vi "Vision_Right_R3.2.vi"() -> ()   [LabVIEW 2015]
uses:
  <vilib>/vision/Pattern Matching.llb/IMAQ Curve Parameters.ctl
  <vilib>/vision/Pattern Matching.llb/IMAQ Match Range Setting.ctl
  <vilib>/userdefined/High Color/IMAQdx.ctl
  <vilib>/vision/driver/NI_Vision_Acquisition_Software.lvlib
  <vilib>/vision/NI_Vision_Development_Module.lvlib
panel:
  in  "Range 0 Default\nSetting Values":T1={"Min Scale"=50.0, "Max Scale"=160.0, "Min Score"=850.0, "Lower Transition Scale"=70.0, "Upper Transition Scale"=200.0, "ROI Vertical"=2.0, "ROI Horizontal"=1.0, "Scale Cushion"=7.0, "Curve Parameters"={"Min Length"=20, "Row Search Step"=15, "Col Search Step"=15}, "Beacon Cushion (px)"=3.0, "Max Scale Diff\nfrom Main"=50.0}
  in  "Range 0 Templates":T2={"Sub - 2 File Path"=path "/home/lvuser/Beacon_Templates/Range_0/Range 0.png", "Sub Beacon Template File Path - ARRAY"=[path "/home/lvuser/Beacon_Templates/Range_1/Sub 0 - Range 1.png", path "/home/lvuser/Beacon_Templates/Range_1/Sub 1 - Range 1.png", path "/home/lvuser/Beacon_Templates/Range_1/Sub 2 - Range 1.png", path "/home/lvuser/Beacon_Templates/Range_1/Sub 3 - Range 1.png", path "/home/lvuser/Beacon_Templates/Range_1/Sub 4 - Range 1.png"]}
  in  "Correlation Score Threhsold (Range 0)":sgl=750.0
  in  "stop":bool
  in  "select (true= use advanced features\nfase= dont use)":bool
  in  "Range 3 Default\nSetting Values":T1={"Min Scale"=50.0, "Max Scale"=130.0, "Min Score"=800.0, "Lower Transition Scale"=1.0, "Upper Transition Scale"=120.0, "ROI Vertical"=4.5, "ROI Horizontal"=2.5, "Scale Cushion"=15.0, "Curve Parameters"={"Min Length"=2, "Row Search Step"=5, "Col Search Step"=5}, "Beacon Cushion (px)"=3.0, "Max Scale Diff\nfrom Main"=10.0}
  in  "Range 2 Default\nSetting Values":T1={"Min Scale"=75.0, "Max Scale"=130.0, "Min Score"=800.0, "Lower Transition Scale"=70.0, "Upper Transition Scale"=115.0, "ROI Vertical"=2.8, "ROI Horizontal"=4.0, "Scale Cushion"=17.0, "Curve Parameters"={"Min Length"=10, "Row Search Step"=10, "Col Search Step"=10}, "Beacon Cushion (px)"=7.0, "Max Scale Diff\nfrom Main"=20.0}
  in  "No Lock Default\nSetting Values":T3={"Min Scale"=25.0, "Max Scale"=125.0, "Min Score"=750.0, "Lower Transition Scale"=35.0, "Upper Transition Scale"=250.0, "ROI Vertical"=15.0, "ROI Horizontal"=15.0, "Scale Cushion"=15.0, "Curve Parameters"={"Min Length"=5, "Row Search Step"=10, "Col Search Step"=10}, "Scale Cushion 2"=15.0, "Max Scale Diff\nfrom Main"=15.0}
  in  "ROI Decay Factor (px)":dbl=50.0
  in  "ROBOT STATE\n(fwd, bwd, neither) 2":i32
  in  "Score Decay \nFactor 2":dbl=50.0
  in  "Range 1 Default\nSetting Values":T1={"Min Scale"=30.0, "Max Scale"=100.0, "Min Score"=800.0, "Lower Transition Scale"=35.0, "Upper Transition Scale"=250.0, "ROI Vertical"=0.75, "ROI Horizontal"=5.0, "Scale Cushion"=20.0, "Curve Parameters"={"Min Length"=15, "Row Search Step"=15, "Col Search Step"=15}, "Beacon Cushion (px)"=25.0, "Max Scale Diff\nfrom Main"=25.0}
  out "Next Template":T4(ring)
  out "Current Template":T4(ring)
  in  "Initial Template":T4(ring)
  in  "Range 3 Templates":T2={"Sub - 2 File Path"=path "/home/lvuser/Beacon_Templates/Range_3/5 Beacons - Range 3.png", "Sub Beacon Template File Path - ARRAY"=[path "/home/lvuser/Beacon_Templates/Range_3/Sub 0 - Range 3.png", path "/home/lvuser/Beacon_Templates/Range_3/Sub 1 - Range 3.png", path "/home/lvuser/Beacon_Templates/Range_3/Sub 2 - Range 3.png", path "/home/lvuser/Beacon_Templates/Range_3/Sub 3 - Range 3.png", path "/home/lvuser/Beacon_Templates/Range_3/Sub 4 - Range 3.png"]}
  in  "Range 2 Templates":T2={"Sub - 2 File Path"=path "/home/lvuser/Beacon_Templates/Range_2/5 Beacons - Range 2.png", "Sub Beacon Template File Path - ARRAY"=[path "/home/lvuser/Beacon_Templates/Range_2/Sub 0 - Range 2.png", path "/home/lvuser/Beacon_Templates/Range_2/Sub 1 - Range 2.png", path "/home/lvuser/Beacon_Templates/Range_2/Sub 2 - Range 2.png", path "/home/lvuser/Beacon_Templates/Range_2/Sub 3 - Range 2.png", path "/home/lvuser/Beacon_Templates/Range_2/Sub 4 - Range 2.png"]}
  in  "Range 1 Templates - LEFT":T2={"Sub - 2 File Path"=path "/home/lvuser/Beacon_Templates/Range_1/2_Beacons_Right - Range 1.png", "Sub Beacon Template File Path - ARRAY"=[path "/home/lvuser/Beacon_Templates/Range_1/Sub 0 - Range 1.png", path "/home/lvuser/Beacon_Templates/Range_1/Sub 1 - Range 1.png", path "/home/lvuser/Beacon_Templates/Range_1/Sub 2 - Range 1.png", path "/home/lvuser/Beacon_Templates/Range_1/Sub 3 - Range 1.png", path "/home/lvuser/Beacon_Templates/Range_1/Sub 4 - Range 1.png"]}
  out "Current Correlation Score":sgl=697.46326
  in  "Correlation Score Threhsold":sgl=300.0
  out "New Min Score":dbl=767.3556925455729
  out "New Low Scale":dbl=92.1760737101237
  out "New high Scale":dbl=122.1760737101237
  in  "Absolute\nMinimum Score":dbl=750.0
  in  "Absolute\nMaximum Scale":dbl=250.0
  in  "Absolute\nMinimum Scale":dbl=25.0
  in  "Score\nCushion":dbl=192.0
  in  "Avg Scale - Last":dbl=107.1760737101237
  in  "Avg Score - Last":dbl=959.3556925455729
  in  "Max Window\n for Avg":u8=3
  in  "Valid Treshold\nfor Lock":i16=3
  out "Current  Score":sgl=956.6209
  out "Current  Scale":sgl=107.15872
  out "Current Valid?":bool=TRUE
  out "Beacon - Scales":sgl[](array[numeric])=[106.93824, 100.57165, 104.69414, 100.46582, 110.0]
  out "beacon - Scores":sgl[](array[numeric])=[992.1048, 981.1018, 1000.0, 999.00995, 773.5499]
  out "Beacons Found":bool[](array[boolean])=[TRUE, TRUE, TRUE, TRUE, TRUE]
  in  "Horiztonall Beacon \nCushion (pixels)":sgl=7.0
  out "Tracking Info":T5={"Lock"=TRUE, "Current Valid"=TRUE, "Current Template"=enum."Range 2", "Tracking Coordinates"={"X"=158.2768096923828, "Y"=119.25008392333984}, "Setting Values"={"Min Score"=767.3556925455729, "Min Scale"=92.1760737101237, "Max Scale"=122.1760737101237, "Curve Parameters"={"Min Length"=10, "Row Search Step"=10, "Col Search Step"=10}}}
  out "dT":u32=420
  out "Avg Scale":dbl=107.1760737101237
  out "Avg Score":dbl=959.3556925455729
  out "Current Search Settings":T8={"Curve Parameters"={"Extraction Mode"=1, "Edge Threshold"=200, "Edge Filter Size"=0, "Min Length"=10, "Row Search Step Size"=10, "Col Search Step Size"=10, "Max Endpoint Gap"=4, "Closed"=TRUE, "Subpixel"=TRUE}, "Match Mode"={"Rotation"=FALSE, "Scale"=TRUE, "Occlusion"=TRUE, "Reserved"=FALSE, "Reserved"=FALSE, "Reserved"=FALSE}, "Range Settings"=[{"Match Constraints"=0, "Min"=-2.0, "Max"=2.0}, {"Match Constraints"=1, "Min"=92.1760737101237, "Max"=122.1760737101237}, {"Match Constraints"=2, "Min"=0.0, "Max"=20.0}], "Number of Matches"=1, "Minimum Match Score"=767.3557, "SubPixel Accuracy"=TRUE, "Adv. Geometric Match Options 2"=[{"Setup Data Item"=20, "Item Value"=0.0}, {"Setup Data Item"=22, "Item Value"=1.0}]} {"Curve Parameters"."Extraction Mode" items=["Normal", "Uniform Regions"]; "Curve Parameters"."Edge Filter Size" items=["Fine", "Normal", "Contour Tracing"]; "Curve Parameters"."Max Endpoint Gap" min=0; "Curve Parameters"."Col Search Step Size" min=1 max=255 step=1; "Curve Parameters"."Row Search Step Size" min=1 max=255 step=1; "Curve Parameters"."Min Length" min=0; "Curve Parameters"."Edge Threshold" min=1 max=350 step=1; "Range Settings"."Max" format="%.2f"; "Range Settings"."Min" format="%.2f"; "Range Settings"."Match Constraints" items=["Rotation Angle (degrees)", "Scale Factor (%)", "Occlusion (%)"]}
  out "Valid Scale History":dbl[](array[numeric])=[107.15872192382812, 107.20863342285156, 107.1608657836914, 106.95974731445312, 107.13298034667969, 106.9737319946289, 107.18673706054688, 106.71354675292969, 106.60578918457031, 106.39472961425781, 106.54171752929688, 105.94715118408203, 107.21797943115234, 106.39393615722656, 106.02467346191406, 106.8507308959961, 106.52826690673828, 105.7506103515625, 107.49342346191406] format="%#_13g"
  out "Valid Score History":dbl[](array[numeric])=[956.6209106445312, 957.1117553710938, 964.3344116210938, 965.7691650390625, 956.08837890625, 958.0139770507812, 954.0676879882812, 955.1304931640625, 955.5637817382812, 955.6036376953125, 955.892822265625, 972.4268798828125, 965.9573974609375, 966.6751098632812, 968.4617309570312, 967.2622680664062, 967.345947265625, 978.3862915039062, 966.6702880859375] format="%#_13g"
  out "Valid Beacon History - in":bool[](array[boolean])=[TRUE, TRUE, TRUE, TRUE, TRUE, TRUE, TRUE, TRUE, TRUE, TRUE, TRUE, TRUE, TRUE, TRUE, TRUE, TRUE, TRUE, TRUE, TRUE]
  out "Startup Flag":bool
  out "Lock Status":bool=TRUE
  out "Y Coordinates":sgl[](array[numeric])=[117.82886, 117.06131, 119.28133, 118.96902, 113.5]
  out "X Coordinates":sgl[](array[numeric])=[55.56325, 105.59997, 158.00548, 202.0866, 251.0]
  out "Right Image out":T9(plugin-control)
  in  "History Size":i32=19
  in  "INITIAL Search Settings":T8={"Curve Parameters"={"Extraction Mode"=1, "Edge Threshold"=200, "Edge Filter Size"=0, "Min Length"=15, "Row Search Step Size"=10, "Col Search Step Size"=10, "Max Endpoint Gap"=4, "Closed"=TRUE, "Subpixel"=TRUE}, "Match Mode"={"Rotation"=TRUE, "Scale"=TRUE, "Occlusion"=TRUE, "Reserved"=FALSE, "Reserved"=FALSE, "Reserved"=FALSE}, "Range Settings"=[{"Match Constraints"=0, "Min"=-10.0, "Max"=1.0}, {"Match Constraints"=1, "Min"=25.0, "Max"=150.0}, {"Match Constraints"=2, "Min"=0.0, "Max"=20.0}], "Number of Matches"=1, "Minimum Match Score"=750.0, "SubPixel Accuracy"=TRUE, "Adv. Geometric Match Options 2"=[{"Setup Data Item"=20, "Item Value"=0.0}, {"Setup Data Item"=22, "Item Value"=1.0}]} {"Curve Parameters"."Extraction Mode" items=["Normal", "Uniform Regions"]; "Curve Parameters"."Edge Filter Size" items=["Fine", "Normal", "Contour Tracing"]; "Curve Parameters"."Max Endpoint Gap" min=0; "Curve Parameters"."Col Search Step Size" min=1 max=255 step=1; "Curve Parameters"."Row Search Step Size" min=1 max=255 step=1; "Curve Parameters"."Min Length" min=0; "Curve Parameters"."Edge Threshold" min=1 max=350 step=1; "Range Settings"."Max" format="%.2f"; "Range Settings"."Min" format="%.2f"; "Range Settings"."Match Constraints" items=["Rotation Angle (degrees)", "Scale Factor (%)", "Occlusion (%)"]; "Adv. Geometric Match Options 2"."Setup Data Item" items=["Curve Extraction Mode", "Curve Edge Threshold", "Curve Edge Filter Size", "Min Curve Length", "Curve Row Search Step Size", "Curve Col Search Step Size", "Curve Max Endpoint Gap", "Extract Closed Curves", "Enable Subpixel Curve Extraction", "Enable Correlation Score", "Enable Subpixel Accuracy", "Subpixel Iterations", "Subpixel Tolerance", "Initial Match List Length", "Enable Target Template Curve Score", "Min Match Separation Distance", "Min Match Separation Angle", "Min Match Separation Scale", "Max Match Overlap", "Enable Coarse Result", "Enable Calibration Support", "Enable Contrast Reversal", "Search Strategy", "Refinement Match Factor", "Subpixel Match Factor"]}
  # "ROI Factore (per Template)"
  # "Template Transition Scales"
  # "Search Parameter Limits"
  # "TEMPLATE FILE PATHS"
  # "Config"
  # "Initial Settings"
  # "Range"
  # "Range"
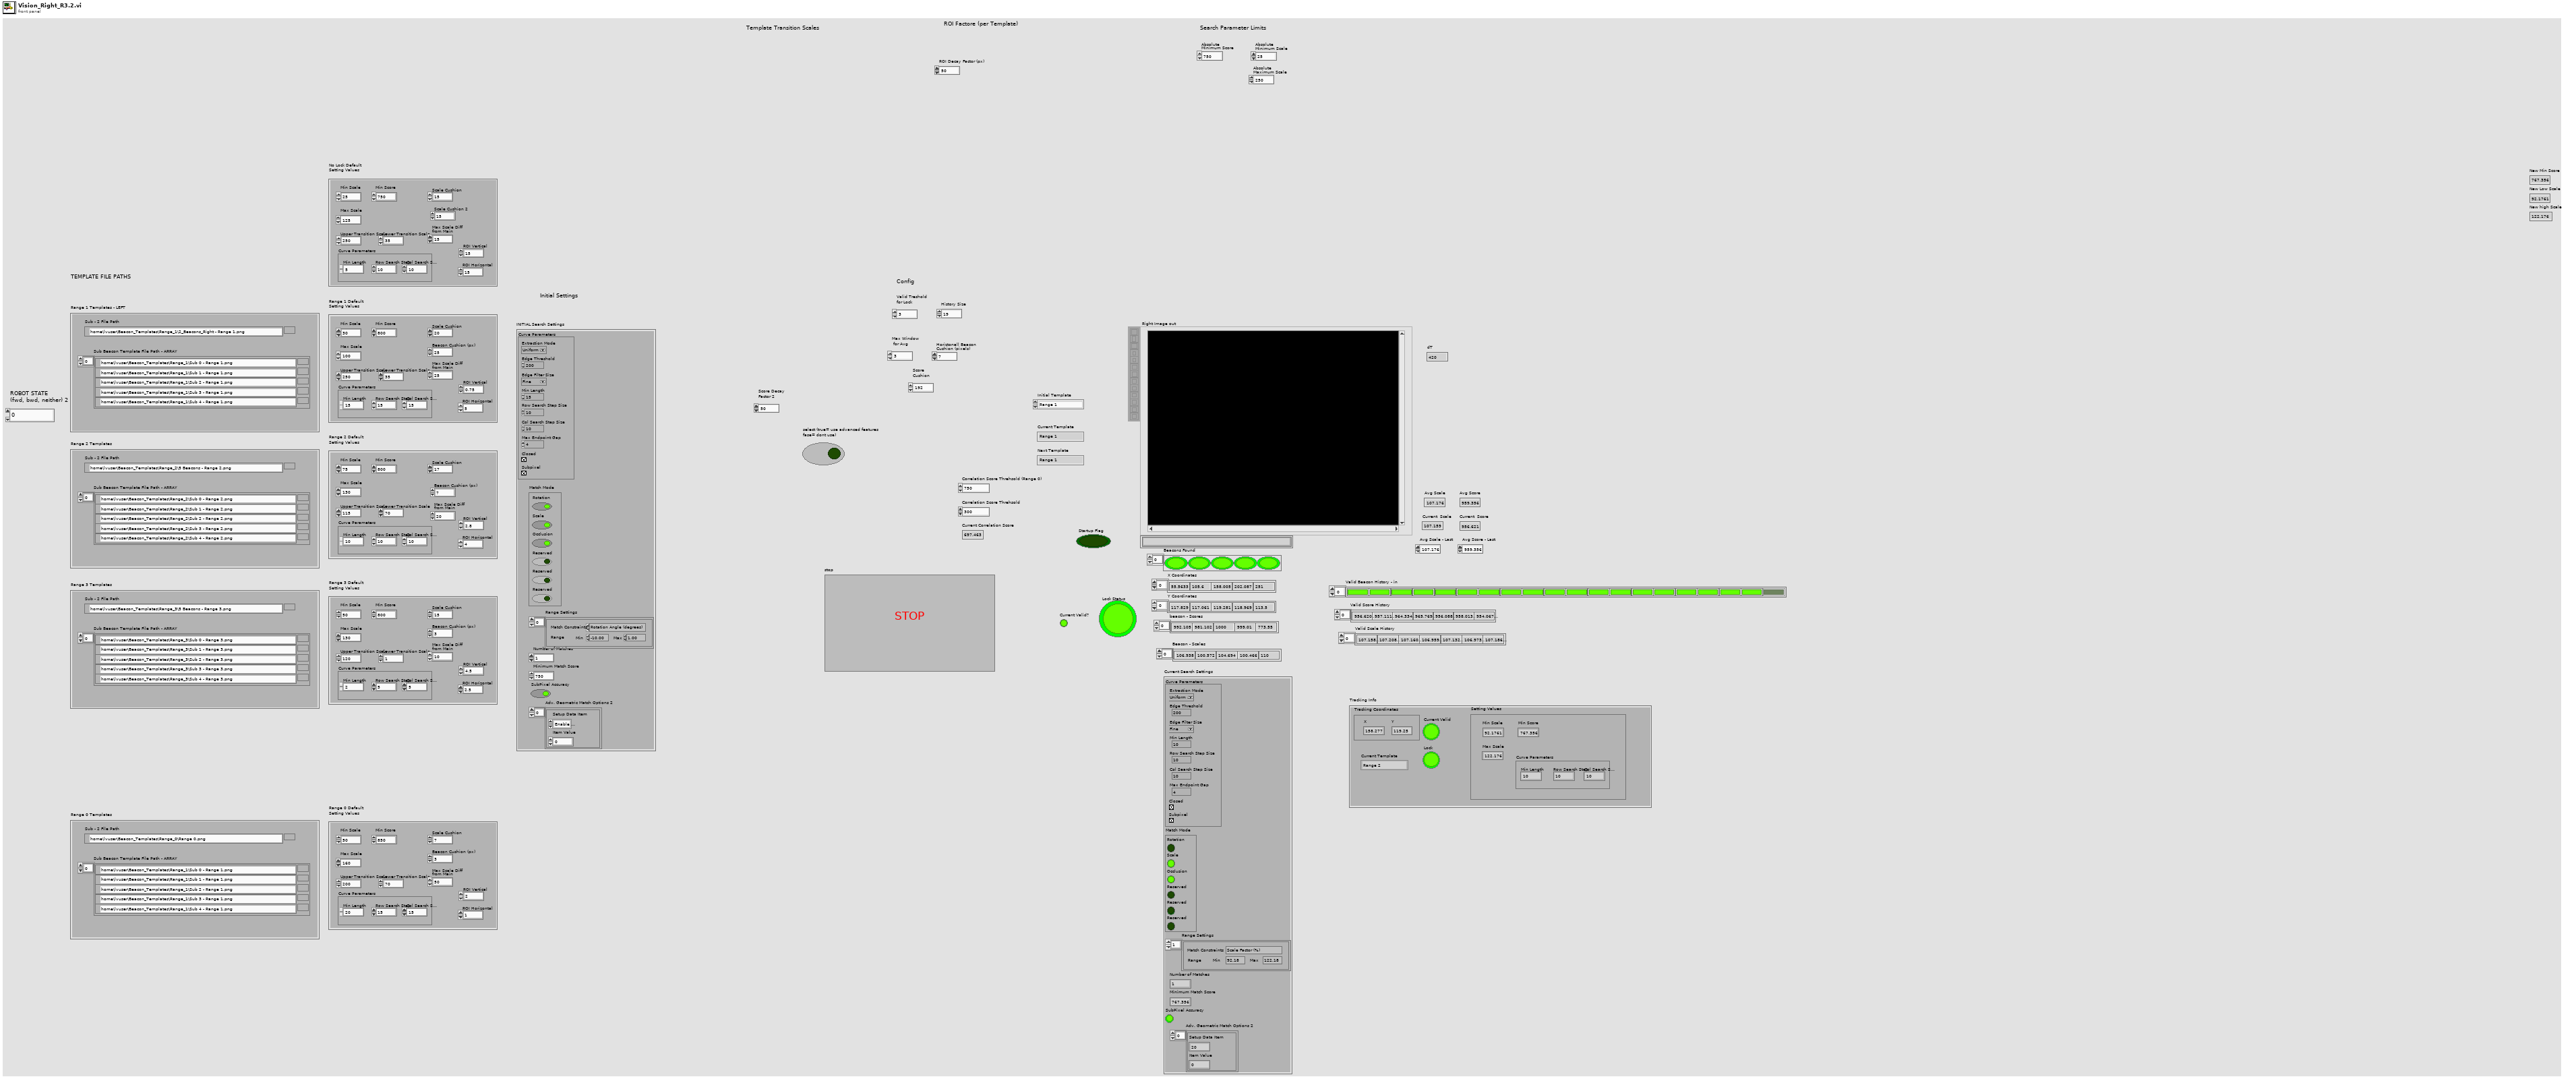
[diagram p1: front panel]
types:
  T1 = cluster{"Min Scale":dbl, "Max Scale":dbl, "Min Score":dbl, "Lower Transition Scale":sgl, "Upper Transition Scale":sgl, "ROI Vertical":dbl, "ROI Horizontal":dbl, "Scale Cushion":dbl, "Curve Parameters":cluster{"Min Length":i32, "Row Search Step":i32, "Col Search Step":i32}, "Beacon Cushion (px)":dbl, "Max Scale Diff\nfrom Main":dbl}
  T2 = cluster{"Sub - 2 File Path":path, "Sub Beacon Template File Path - ARRAY":path[]}
  T3 = cluster{"Min Scale":dbl, "Max Scale":dbl, "Min Score":dbl, "Lower Transition Scale":sgl, "Upper Transition Scale":sgl, "ROI Vertical":dbl, "ROI Horizontal":dbl, "Scale Cushion":dbl, "Curve Parameters":cluster{"Min Length":i32, "Row Search Step":i32, "Col Search Step":i32}, "Scale Cushion 2":dbl, "Max Scale Diff\nfrom Main":dbl}
  T4 = enum16{"Range 1", "Range 2", "Range 3", "Range 0"}
  T5 = cluster{"Lock":bool, "Current Valid":bool, "Current Template":enum16{"Range 1", "Range 2", "Range 3", "Range 0"}, "Tracking Coordinates":cluster{"X":dbl, "Y":dbl}, "Setting Values":cluster{"Min Score":dbl, "Min Scale":dbl, "Max Scale":dbl, "Curve Parameters":cluster{"Min Length":i32, "Row Search Step":i32, "Col Search Step":i32}}}
  T6 = typedef "IMAQ Curve Parameters.ctl" = cluster{"Extraction Mode":u32, "Edge Threshold":i32, "Edge Filter Size":u32, "Min Length":i32, "Row Search Step Size":i32, "Col Search Step Size":i32, "Max Endpoint Gap":i32, "Closed":bool, "Subpixel":bool}
  T7 = typedef "IMAQ Match Range Setting.ctl" = cluster{"Match Constraints":u32, "Min":dbl, "Max":dbl}
  T8 = cluster{"Curve Parameters":T6, "Match Mode":cluster{"Rotation":bool, "Scale":bool, "Occlusion":bool, "Reserved":bool, "Reserved":bool, "Reserved":bool}, "Range Settings":T7[], "Number of Matches":i32, "Minimum Match Score":sgl, "SubPixel Accuracy":bool, "Adv. Geometric Match Options 2":cluster{"Setup Data Item":u16, "Item Value":dbl}[]}
  T9 = typedef "IMAQ Image.ctl" = refnum<image>
  T10 = typedef "IMAQdx.ctl" = refnum<k21>
  T11 = typedef "Image Type" = u32
  T12 = typedef "ROI Descriptor" = cluster{"Global Rectangle":i32[], "Contours":cluster{"ID":enum32{"External", "Internal"}, "Type":u32, "Coordinates":i32[]}[]}
  T13 = typedef "IMAQ GM Match Report.ctl" = cluster{"Position":cluster{"x":sgl, "y":sgl}, "Angle":sgl, "Scale":sgl, "Score":sgl, "Bounding Box":cluster{"x":sgl, "y":sgl}[], "Contrast Reversed":bool, "Occlusion %":sgl, "Template Target Curve Score":sgl, "Target Template Curve Score":sgl, "Correlation Score":sgl}
  T14 = cluster{"Matches[0]":T13, "Matches[1]":T13, "Matches[2]":T13, "Matches[3]":T13, "Matches[4]":T13, "Matches[5]":T13, "Matches[6]":T13, "Matches[7]":T13, "Matches[8]":T13}
  T15 = cluster{"Bounding Box[0]":cluster{"x":sgl, "y":sgl}, "Bounding Box[1]":cluster{"x":sgl, "y":sgl}, "Bounding Box[2]":cluster{"x":sgl, "y":sgl}, "Bounding Box[3]":cluster{"x":sgl, "y":sgl}, "Bounding Box[4]":cluster{"x":sgl, "y":sgl}, "Bounding Box[5]":cluster{"x":sgl, "y":sgl}, "Bounding Box[6]":cluster{"x":sgl, "y":sgl}, "Bounding Box[7]":cluster{"x":sgl, "y":sgl}, "Bounding Box[8]":cluster{"x":sgl, "y":sgl}}
  T16 = cluster{"Matches (Geometric Matching 1)[0]":T13, "Matches (Geometric Matching 1)[1]":T13, "Matches (Geometric Matching 1)[2]":T13, "Matches (Geometric Matching 1)[3]":T13, "Matches (Geometric Matching 1)[4]":T13, "Matches (Geometric Matching 1)[5]":T13, "Matches (Geometric Matching 1)[6]":T13, "Matches (Geometric Matching 1)[7]":T13, "Matches (Geometric Matching 1)[8]":T13}
  T17 = cluster{"Min Length":i32, "Row Search Step":i32, "Col Search Step":i32}
  T18 = cluster{"Extraction Mode":u32, "Edge Threshold":i32, "Edge Filter Size":u32, "Min Length":i32, "Row Search Step":i32, "Col Search Step":i32, "Max Endpoint Gap":i32, "Closed":bool, "Subpixel":bool}
  T19 = typedef "IMAQ Rectangle" = cluster{"Left":i32, "Top":i32, "Right":i32, "Bottom":i32, "Rotation":dbl}
  T20 = cluster{"Min Length":i32, "Row Search Step Size":i32, "Col Search Step Size":i32}
  T21 = cluster{"Min Score":dbl, "Min":dbl, "Max":dbl, cluster{"Min Length":i32, "Row Search Step Size":i32, "Col Search Step Size":i32}}
  T22 = cluster{bool, bool, "Initial Template":enum16{"Range 1", "Range 2", "Range 3", "Range 0"}, "Position":cluster{"x":dbl, "y":dbl}, cluster{"Min Score":dbl, "Min":dbl, "Max":dbl, cluster{"Min Length":i32, "Row Search Step Size":i32, "Col Search Step Size":i32}}}
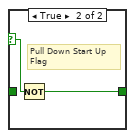
[diagram p2: hidden frame]
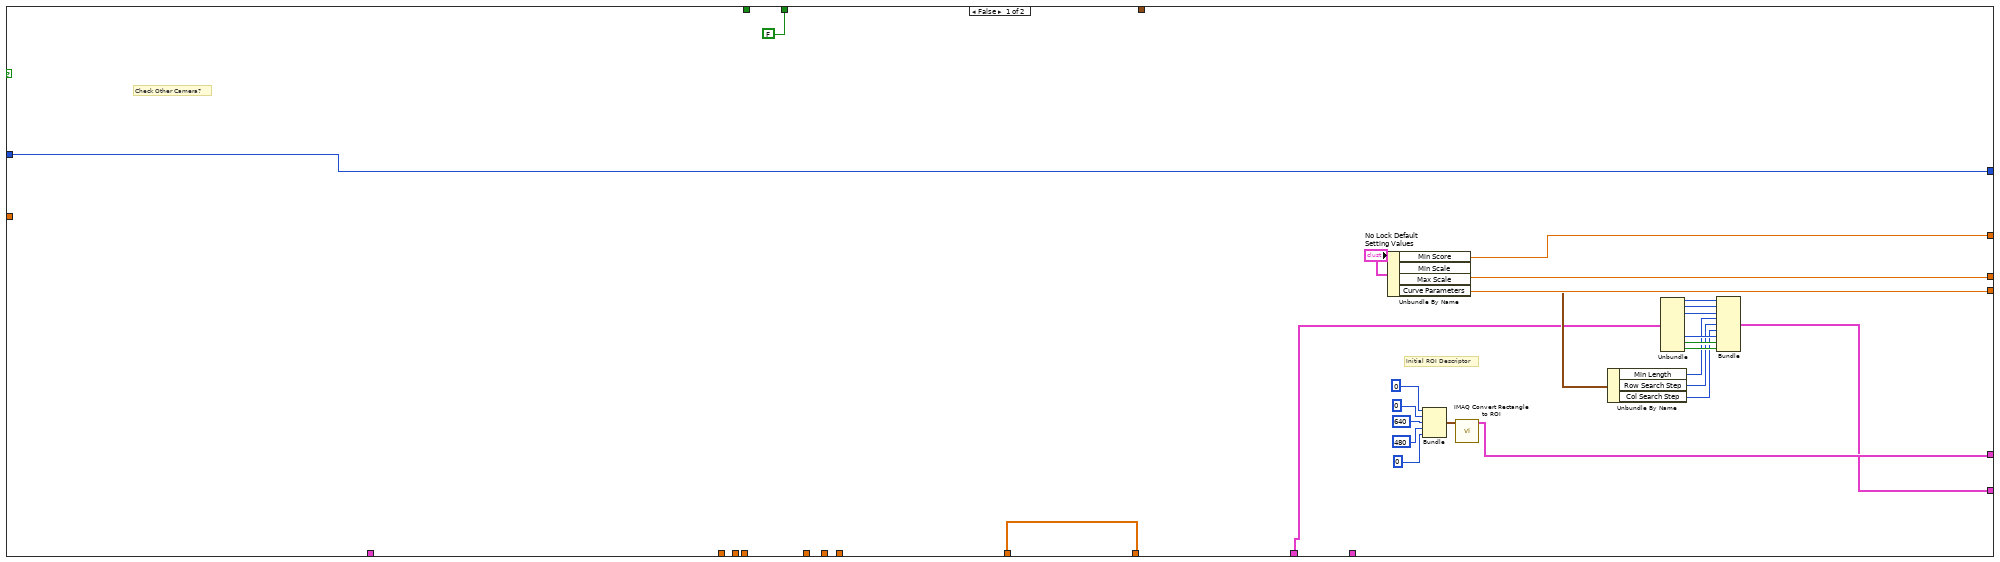
[diagram p3: hidden frame]
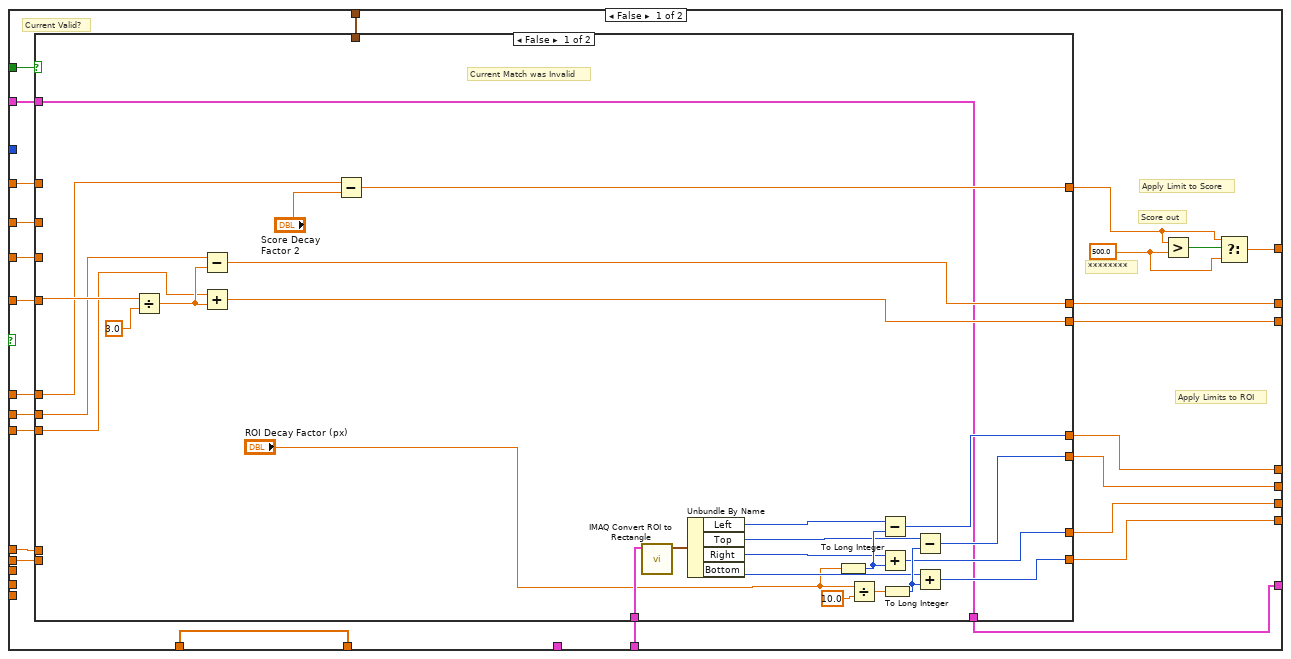
[diagram p4: hidden frame]
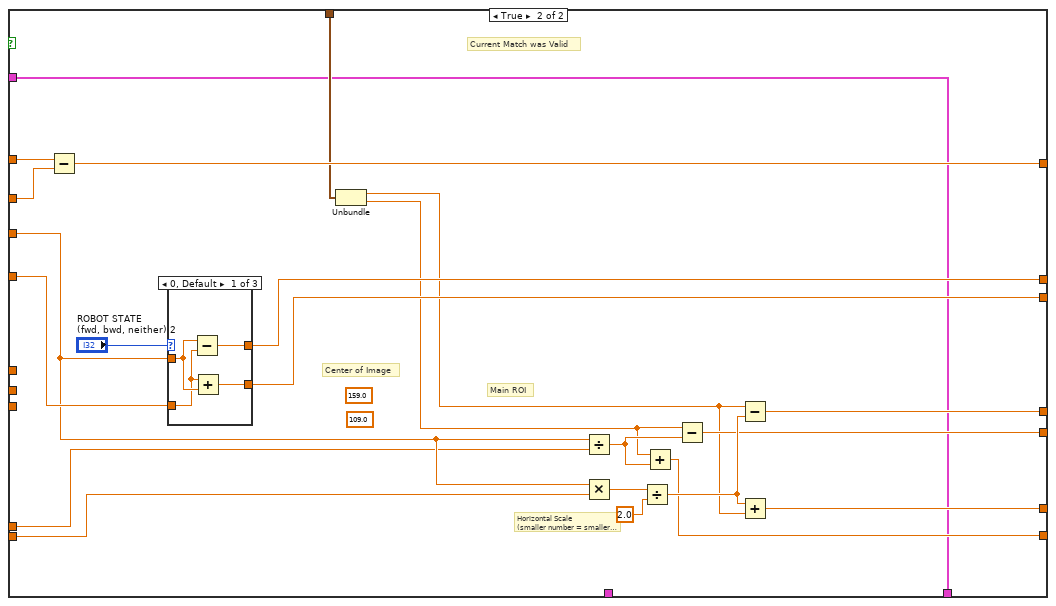
[diagram p5: hidden frame]
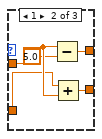
[diagram p6: hidden frame]
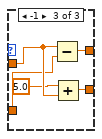
[diagram p7: hidden frame]
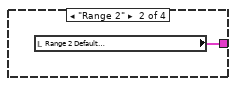
[diagram p8: hidden frame]
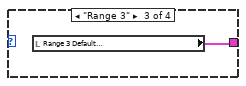
[diagram p9: hidden frame]
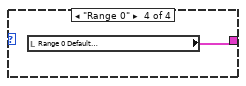
[diagram p10: hidden frame]
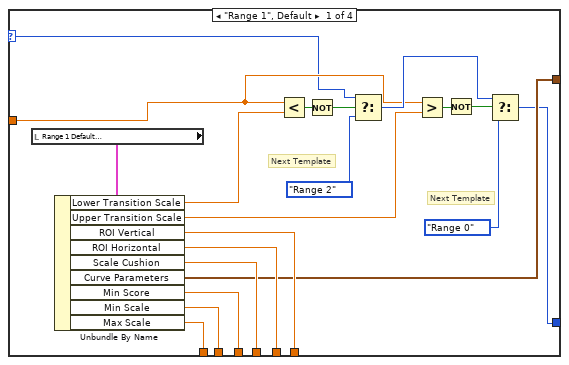
[diagram p11: hidden frame]
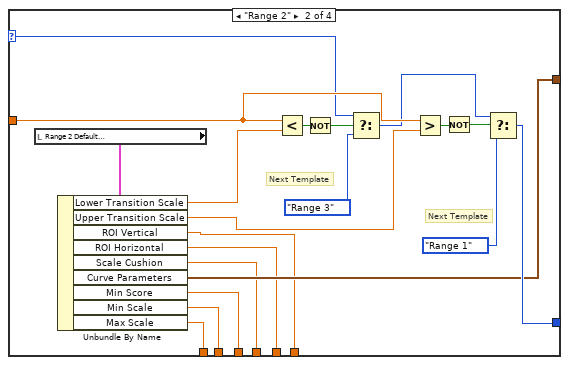
[diagram p12: hidden frame]
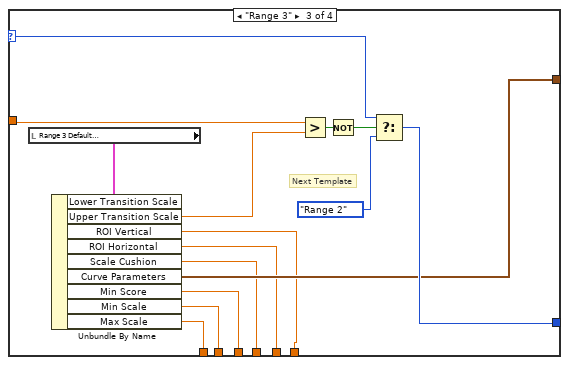
[diagram p13: hidden frame]
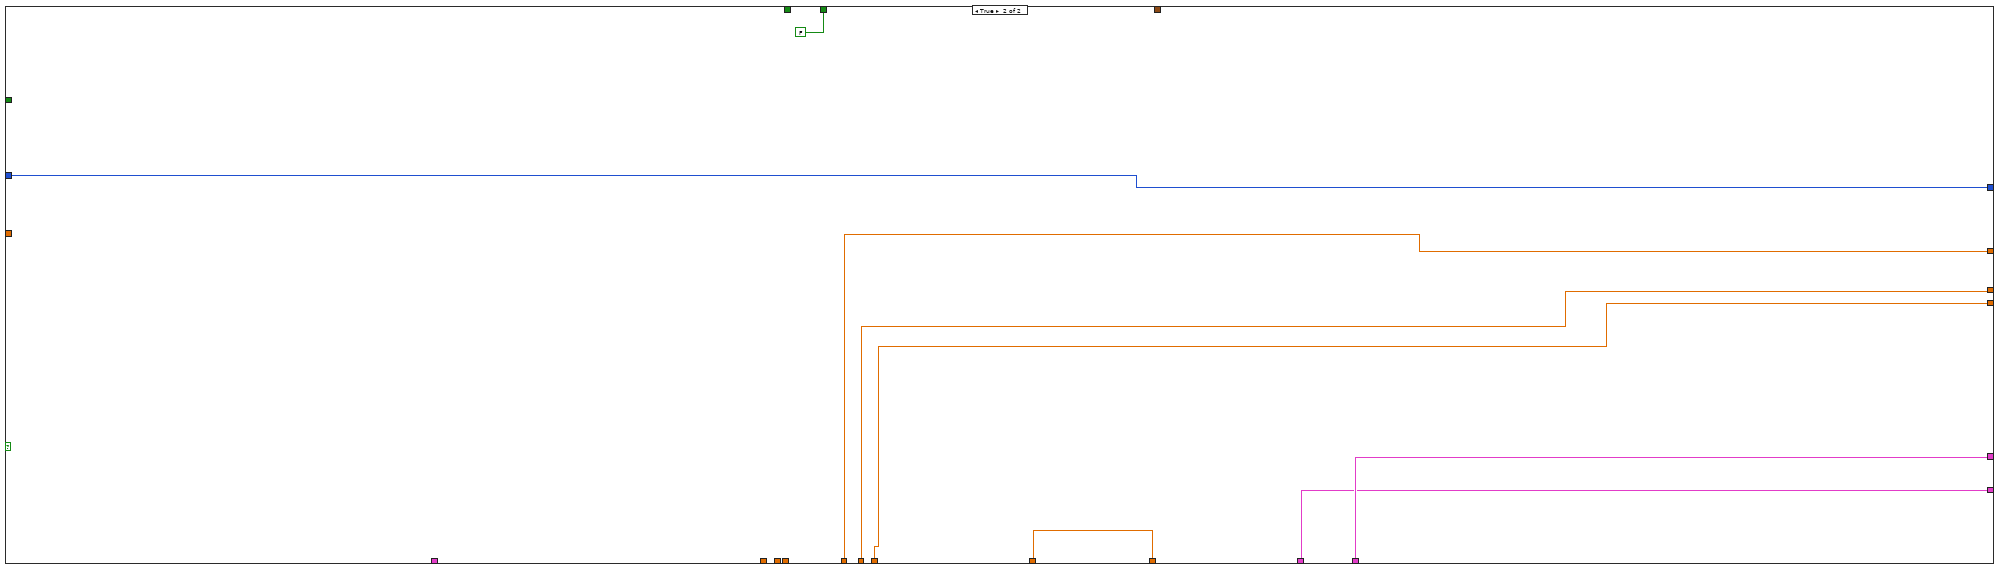
[diagram p14: hidden frame]
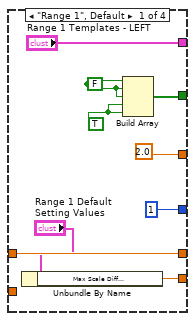
[diagram p15: hidden frame]
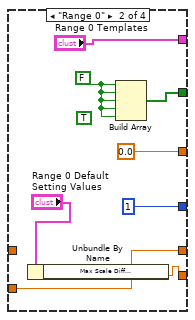
[diagram p16: hidden frame]
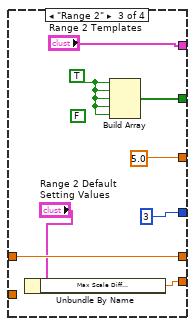
[diagram p17: hidden frame]
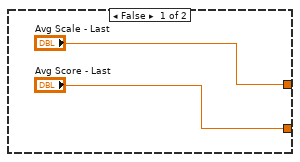
[diagram p18: hidden frame]
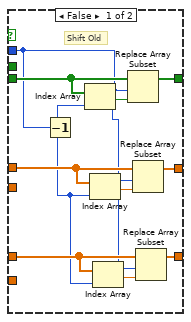
[diagram p20: hidden frame]
diagram:
  n1 = flat-sequence {
    tunnel: [w38] -> w16
    tunnel: ["INITIAL Search Settings"] -> w15
    tunnel: ["Initial Template"] -> w14
    tunnel: [TRUE] -> w13
    tunnel: [w35] -> w12
    tunnel: [w34] -> w11
    tunnel: [w33] -> w10
    tunnel: [w32] -> w9
    tunnel: [w31] -> w8
    tunnel: ["History Size"] -> w7
    tunnel: [750.0] -> w6
    tunnel: [100.0] -> w5
    tunnel: [w19] -> w4
    tunnel: [w18] -> w3
    tunnel: [w17] -> w2
    tunnel: w16 -> [w64]
    tunnel: w15 -> [w63]
    tunnel: w14 -> [w62]
    tunnel: w13 -> [w61]
    tunnel: w12 -> [w57]
    tunnel: w11 -> [w54]
    tunnel: w10 -> [w60]
    tunnel: w9 -> [w59]
    tunnel: w8 -> [w58]
    tunnel: w7 -> [w56]
    tunnel: w6 -> [_]
    tunnel: w5 -> [_]
    tunnel: w4 -> [w53]
    tunnel: w3 -> [w52]
    tunnel: w2 -> [w51]
    tunnel: [w50] -> w1
    tunnel: w1 -> [w825]
    frame #0 {
      w24 = "[NIIMAQ_HEADER]\nType = 2\nVersion = 8\n\n[CAMERA_DATA]\nAcquisitionAttributes::Bayer::Algorithm = \"Bilinear\"\nAcquisitionAttributes::Bayer::GainB = \"1\"\nAcquisitionAttributes::Bayer::GainG = \"1\"\nAcquisitionAttributes::Bayer::GainR = \"1\"\nAcquisitionAttributes::Bayer::Pattern = \"Use hardware value\"\nAcquisitionAttributes::BitsPerPixel = \"Use hardware value\"\nAcquisitionAttributes::IgnoreFirstFrame = \"false\"\nAcquisitionAttributes::ImageDecoderCopyMode = \"Auto\"\nAcquisitionAttributes::OutputImageType = \"Auto\"\nAcquisitionAttributes::OverwriteMode = \"Get Newest\"\nAcquisitionAttributes::PixelSignedness = \"Use hardware value\"\nAcquisitionAttributes::ReceiveTimestampMode = \"None\"\nAcquisitionAttributes::ShiftPixelBits = \"false\"\nAcquisitionAttributes::SwapPixelBytes = \"false\"\nAcquisitionAttributes::Timeout = \"5000\"\nAcquisitionAttributes::VerticalMirror = \"false\"\nAcquisitionAttributes::VideoMode = \"320x240 YUY2 30.00fps\"\nCameraAttributes::BacklightCompensation::Mode = \"Manual\"\nCameraAttributes::BacklightCompensation::Value = \"false\"\nCameraAttributes::Brightness::Mode = \"UnknownEnumValue\"\nCameraAttributes::Brightness::Value = \"133\"\nCameraAttributes::Contrast::Mode = \"Manual\"\nCameraAttributes::Contrast::Value = \"0\"\nCameraAttributes::Exposure::Mode = \"Auto\"\nCameraAttributes::Focus::Mode = \"Auto\"\nCameraAttributes::Pan::Mode = \"Manual\"\nCameraAttributes::Pan::Value = \"0\"\nCameraAttributes::Saturation::Mode = \"Manual\"\nCameraAttributes::Saturation::Value = \"103\"\nCameraAttributes::Sharpness::Mode = \"Manual\"\nCameraAttributes::Sharpness::Value = \"25\"\nCameraAttributes::Tilt::Mode = \"Manual\"\nCameraAttributes::Tilt::Value = \"0\"\nCameraAttributes::WhiteBalance::Mode = \"Auto\"\nCameraAttributes::Zoom::Mode = \"Manual\"\nCameraAttributes::Zoom::Value = \"0\"\n"  # Attributes
      w45 = T11 0 items=["Grayscale (U8)", "Grayscale (I16)", "Grayscale (SGL)", "Complex (CSG)", "RGB (U32)", "HSL (U32)", "RGB (U64)", "Grayscale (U16)"] ("Image Type")
      # "avg start scale"
      # "Score History"
      # "Scale History"
      # "Valid Match History\n(main beacon)"
      # "Template State"
      # "Search Parameters"
      # "StartUp = True"
      # "Initial ROI Descriptor"
      # "INITIALIZE"
      n2 = call <vilib>:"IMAQdx Open Camera.vi"("Session In"=T10 "cam0") -> ("error out"=w22:errorcluster, "Session Out"=w23:T10)  [unwired: 2 in, 7 out]
      n3 = call <vilib>:"IMAQdx Read Attributes From String.vi"("error in"=w22, "Attributes String In"=w24, "Session In"=w23) -> ("error out"=w21:errorcluster, "Session Out"=w20:T10)  [unwired: 7 out]
      n4 = Bundle(0, 0, 640, 480, 0) -> (w44:cluster{i32, i32, i32, i32, i32})  [unwired: 1 in]
      n5 = call "IMAQ Convert Rectangle to ROI"("Rectangle"=w44) -> ("ROI Descriptor"=w38:T12)  [unwired: 8 in, 1 out]
      n6 = call "IMAQ Create"("Image Name"="Left_Image", "Image Type"=w45) -> ("New Image"=w35:T9, "error out"=w34:errorcluster)  [unwired: 3 in]
      n7 = Initialize Array(FALSE, "History Size") -> (w33:bool[])
      n8 = Initialize Array(0.0, "History Size") -> (w31:dbl[])
      n9 = Initialize Array(0.0, "History Size") -> (w32:dbl[])
      n10 = call <vilib>:"IMAQdx Configure Grab.vi"("error in"=w21, "Session In"=w20) -> ("error out"=w17:errorcluster, "Session Out"=w19:T10)  [unwired: 8 in]
      n11 = call "IMAQ Create"("Image Name"="Original") -> ("New Image"=w18:T9)  [unwired: 4 in, 1 out]
    }
    frame #1 {
      # "Avg Scale"
      # "Avg Score"
      # "Score History"
      # "Scale History"
      # "Valid Match History\n(main beacon)"
      # "Sub Beacon Search Array"
      # "StartUp = True"
      # "Template State"
      # "Search Parameters"
      # "ROI"
      n12 = call "Tick Count"() -> ("Tick Count(mSec)"=w55:u32)
      n13 = while {
        shift-right: [w77] -> _
        shift-left: w64 -> [w91]
        shift-right: [w87] -> _
        shift-left: w63 -> [w92]
        shift-right: [w76] -> _
        shift-left: w62 -> [w79]
        shift-right: [w74] -> _
        shift-left: w61 -> [w75]
        shift-right: [w83] -> _
        shift-left: w60 -> [w84]
        shift-right: [w73] -> _
        shift-left: w59 -> [w82]
        shift-right: [w80] -> _
        shift-left: w58 -> [w81]
        shift-right: [w86] -> _
        shift-left: w57 -> [w93]
        tunnel: w56 -> [w98]
        shift-right: [w96] -> _
        shift-left: w55 -> [w97]
        tunnel: w54 -> [w85]
        tunnel: w53 -> [w72]
        tunnel: w52 -> [w71]
        tunnel: w51 -> [w70]
        tunnel: [w67] -> w50
        stop <- "stop" stop-if-true
        n14 = call "Tick Count2"() -> ("Tick Count(mSec)"=w96:u32)
        n15 = Subtract(x=w96, y=w97) -> (x-y=→"dT":u32)
        n16 = flat-sequence {
          tunnel: [w106] -> w89
          tunnel: [w105] -> w94
          tunnel: w93 -> [w105]
          tunnel: [w105] -> w86
          tunnel: w85 -> [_]
          tunnel: w72 -> [w104]
          tunnel: w71 -> [w103]
          tunnel: w70 -> [w102]
          tunnel: [w101] -> w69
          tunnel: [w100] -> w68
          tunnel: [w99] -> w66
          tunnel: w79 -> [w110]
          tunnel: w84 -> [w223]
          tunnel: w82 -> [w222]
          tunnel: w81 -> [w221]
          tunnel: w98 -> [_]
          tunnel: w94 -> [w121]
          tunnel: w92 -> [w122]
          tunnel: w91 -> [w124]
          tunnel: [w190] -> w90
          tunnel: w89 -> [w179]
          tunnel: [w179] -> w88
          tunnel: [w178] -> w83
          tunnel: [w146] -> _
          tunnel: [w177] -> w80
          tunnel: w75 -> [w143]
          tunnel: [w148] -> w78
          tunnel: [w149] -> w77
          tunnel: [w148] -> w76
          tunnel: [w142] -> w74
          tunnel: [w147] -> w73
          tunnel: w69 -> [w116]
          tunnel: w68 -> [w115]
          tunnel: [w114] -> w67
          tunnel: w66 -> [w114]
          tunnel: w90 -> [w822]
          tunnel: w88 -> [w823]
          tunnel: [w822] -> w87
          tunnel: [w821] -> _
          tunnel: w78 -> [w821]
          frame #0 {
            # "Aquire Image"
            n17 = shared-variable "RT myRIO Target - Overlord\\Localization_Variables_r0.lvlib\\Right Servo Angle_Current"() -> (w106:dbl)  [unwired: 1 in, 1 out]
            n18 = call <vilib>:"IMAQdx Grab2.vi"("error in"=w102, "Image In"=w103, "Session In"=w104) -> ("error out"=w100:errorcluster, "Image Out"=w101:T9, "Session Out"=w99:T10)  [unwired: 5 in, 1 out]
          }
          frame #1 {
            (unwired) T4."Range 1" ("Initial Template 2")
            w134 = 6 items=["Red", "Green", "Blue", "Hue", "Saturation", "Luminance", "Value", "Intensity"] ("Color Plane")
            w193 = u32 1 ("index")
            # "Tracking Position"
            # "ROI center"
            # "Add mode when CLose to look for all individual beacons with full ROI"
            # "Service Start Up Flag"
            # "Change States?"
            # "Next Template"
            # "Max Scale"
            # "Min Scale"
            # "Min Score"
            # "Curve p"
            # "ROI"
            # "Current Scale Range"
            # "Current Min Score"
            # "Avg Score"
            # "Avg Scale"
            # "Startup?"
            # "********** Look into False case **********"
            # "SUm # of Sub-Beacons Found, Check if Enoough\nto be considered Valid"
            # "Update Tracking Coordinates"
            # "Next Settings"
            # "Current Settings"
            # "Current Min\n& Max Scale"
            # "Scale"
            # "Min Score"
            # "Lower Scale"
            # "Upper Scale"
            # "Min Score out"
            # "Score History"
            # "Min Required to use avarage"
            # "Scale History"
            # "History Size"
            # "Calculate Average Score/Scale"
            # "****# of previous in history that must be true\nin order for position to be considered \"locked\""
            # "Scale History"
            # "Score History"
            # "Valid History"
            # "Update History Data"
            # "1 Match FOund?"
            # "# of Sub Beacons"
            # "Sub Beacons to Search For"
            # "# Sub Beacons to Find in\norder to be valid"
            # "Template Filepath & Sub Beacon Array"
            # "Select Current Template Config"
            # "Pattern Match to Current Template"
            # "Apply FIltering"
            n19 = call "IMAQ ImageBorderSize"("Get/Set Status? (Set)"=TRUE, "Image"=w116, "Image border size in"=13 ("Border Size"), "error in (no error)"=w115) -> ("Image Out"=w133:T9, "error out"=w137:errorcluster)  [unwired: 1 out]
            n20 = call "IMAQ ExtractSingleColorPlane"("Color Plane"=w134, "error in (no error)"=w137, "Image Src"=w133) -> ("error out"=w132:errorcluster, "Image Dst Out"=w130:T9)  [unwired: 1 in, 6 out]
            n21 = call "IMAQ Convolute"("Kernel"=sgl[][] [[1.0, 2.0, 1.0], [2.0, 4.0, 2.0], [1.0, 2.0, 1.0]], "Divider (kernel sum)"=sgl 9.0 ("Divider"), "error in (no error)"=w132, "Image Src"=w130) -> ("error out"=w129:errorcluster, "Image Dst Out"=w126:T9)  [unwired: 3 in, 3 out]
            n22 = call "IMAQ Convolute"("Kernel"=sgl[][] [[-1.0, -1.0, -1.0, -1.0, -1.0, -1.0, -1.0, -1.0, -1.0, -1.0, -1.0, -1.0, -1.0, -1.0, -1.0, -1.0, -1.0, -1.0, -1.0, -1.0, -1.0, -1.0, -1.0, -1.0, -1.0, -1.0, -1.0], [-1.0, -1.0, -1.0, -1.0, -1.0, -1.0, -1.0, -1.0, -1.0, -1.0, -1.0, -1.0, -1.0, -1.0, -1.0, -1.0, -1.0, -1.0, -1.0, -1.0, -1.0, -1.0, -1.0, -1.0, -1.0, -1.0, -1.0], [-1.0, -1.0, -1.0, -1.0, -1.0, -1.0, -1.0, -1.0, -1.0, -1.0, -1.0, -1.0, -1.0, -1.0, -1.0, -1.0, -1.0, -1.0, -1.0, -1.0, -1.0, -1.0, -1.0, -1.0, -1.0, -1.0, -1.0], [-1.0, -1.0, -1.0, -1.0, -1.0, -1.0, -1.0, -1.0, -1.0, -1.0, -1.0, -1.0, -1.0, -1.0, -1.0, -1.0, -1.0, -1.0, -1.0, -1.0, -1.0, -1.0, -1.0, -1.0, -1.0, -1.0, -1.0], [-1.0, -1.0, -1.0, -1.0, -1.0, -1.0, -1.0, -1.0, -1.0, -1.0, -1.0, -1.0, -1.0, -1.0, -1.0, -1.0, -1.0, -1.0, -1.0, -1.0, -1.0, -1.0, -1.0, -1.0, -1.0, -1.0, -1.0], [-1.0, -1.0, -1.0, -1.0, -1.0, -1.0, -1.0, -1.0, -1.0, -1.0, -1.0, -1.0, -1.0, -1.0, -1.0, -1.0, -1.0, -1.0, -1.0, -1.0, -1.0, -1.0, -1.0, -1.0, -1.0, -1.0, -1.0], [-1.0, -1.0, -1.0, -1.0, -1.0, -1.0, -1.0, -1.0, -1.0, -1.0, -1.0, -1.0, -1.0, -1.0, -1.0, -1.0, -1.0, -1.0, -1.0, -1.0, -1.0, -1.0, -1.0, -1.0, -1.0, -1.0, -1.0], [-1.0, -1.0, -1.0, -1.0, -1.0, -1.0, -1.0, -1.0, -1.0, -1.0, -1.0, -1.0, -1.0, -1.0, -1.0, -1.0, -1.0, -1.0, -1.0, -1.0, -1.0, -1.0, -1.0, -1.0, -1.0, -1.0, -1.0], [-1.0, -1.0, -1.0, -1.0, -1.0, -1.0, -1.0, -1.0, -1.0, -1.0, -1.0, -1.0, -1.0, -1.0, -1.0, -1.0, -1.0, -1.0, -1.0, -1.0, -1.0, -1.0, -1.0, -1.0, -1.0, -1.0, -1.0], [-1.0, -1.0, -1.0, -1.0, -1.0, -1.0, -1.0, -1.0, -1.0, -1.0, -1.0, -1.0, -1.0, -1.0, -1.0, -1.0, -1.0, -1.0, -1.0, -1.0, -1.0, -1.0, -1.0, -1.0, -1.0, -1.0, -1.0], [-1.0, -1.0, -1.0, -1.0, -1.0, -1.0, -1.0, -1.0, -1.0, -1.0, -1.0, -1.0, -1.0, -1.0, -1.0, -1.0, -1.0, -1.0, -1.0, -1.0, -1.0, -1.0, -1.0, -1.0, -1.0, -1.0, -1.0], [-1.0, -1.0, -1.0, -1.0, -1.0, -1.0, -1.0, -1.0, -1.0, -1.0, -1.0, -1.0, -1.0, -1.0, -1.0, -1.0, -1.0, -1.0, -1.0, -1.0, -1.0, -1.0, -1.0, -1.0, -1.0, -1.0, -1.0], [-1.0, -1.0, -1.0, -1.0, -1.0, -1.0, -1.0, -1.0, -1.0, -1.0, -1.0, -1.0, -1.0, -1.0, -1.0, -1.0, -1.0, -1.0, -1.0, -1.0, -1.0, -1.0, -1.0, -1.0, -1.0, -1.0, -1.0], [-1.0, -1.0, -1.0, -1.0, -1.0, -1.0, -1.0, -1.0, -1.0, -1.0, -1.0, -1.0, -1.0, 728.0, -1.0, -1.0, -1.0, -1.0, -1.0, -1.0, -1.0, -1.0, -1.0, -1.0, -1.0, -1.0, -1.0], [-1.0, -1.0, -1.0, -1.0, -1.0, -1.0, -1.0, -1.0, -1.0, -1.0, -1.0, -1.0, -1.0, -1.0, -1.0, -1.0, -1.0, -1.0, -1.0, -1.0, -1.0, -1.0, -1.0, -1.0, -1.0, -1.0, -1.0], [-1.0, -1.0, -1.0, -1.0, -1.0, -1.0, -1.0, -1.0, -1.0, -1.0, -1.0, -1.0, -1.0, -1.0, -1.0, -1.0, -1.0, -1.0, -1.0, -1.0, -1.0, -1.0, -1.0, -1.0, -1.0, -1.0, -1.0], [-1.0, -1.0, -1.0, -1.0, -1.0, -1.0, -1.0, -1.0, -1.0, -1.0, -1.0, -1.0, -1.0, -1.0, -1.0, -1.0, -1.0, -1.0, -1.0, -1.0, -1.0, -1.0, -1.0, -1.0, -1.0, -1.0, -1.0], [-1.0, -1.0, -1.0, -1.0, -1.0, -1.0, -1.0, -1.0, -1.0, -1.0, -1.0, -1.0, -1.0, -1.0, -1.0, -1.0, -1.0, -1.0, -1.0, -1.0, -1.0, -1.0, -1.0, -1.0, -1.0, -1.0, -1.0], [-1.0, -1.0, -1.0, -1.0, -1.0, -1.0, -1.0, -1.0, -1.0, -1.0, -1.0, -1.0, -1.0, -1.0, -1.0, -1.0, -1.0, -1.0, -1.0, -1.0, -1.0, -1.0, -1.0, -1.0, -1.0, -1.0, -1.0], [-1.0, -1.0, -1.0, -1.0, -1.0, -1.0, -1.0, -1.0, -1.0, -1.0, -1.0, -1.0, -1.0, -1.0, -1.0, -1.0, -1.0, -1.0, -1.0, -1.0, -1.0, -1.0, -1.0, -1.0, -1.0, -1.0, -1.0], [-1.0, -1.0, -1.0, -1.0, -1.0, -1.0, -1.0, -1.0, -1.0, -1.0, -1.0, -1.0, -1.0, -1.0, -1.0, -1.0, -1.0, -1.0, -1.0, -1.0, -1.0, -1.0, -1.0, -1.0, -1.0, -1.0, -1.0], [-1.0, -1.0, -1.0, -1.0, -1.0, -1.0, -1.0, -1.0, -1.0, -1.0, -1.0, -1.0, -1.0, -1.0, -1.0, -1.0, -1.0, -1.0, -1.0, -1.0, -1.0, -1.0, -1.0, -1.0, -1.0, -1.0, -1.0], [-1.0, -1.0, -1.0, -1.0, -1.0, -1.0, -1.0, -1.0, -1.0, -1.0, -1.0, -1.0, -1.0, -1.0, -1.0, -1.0, -1.0, -1.0, -1.0, -1.0, -1.0, -1.0, -1.0, -1.0, -1.0, -1.0, -1.0], [-1.0, -1.0, -1.0, -1.0, -1.0, -1.0, -1.0, -1.0, -1.0, -1.0, -1.0, -1.0, -1.0, -1.0, -1.0, -1.0, -1.0, -1.0, -1.0, -1.0, -1.0, -1.0, -1.0, -1.0, -1.0, -1.0, -1.0], [-1.0, -1.0, -1.0, -1.0, -1.0, -1.0, -1.0, -1.0, -1.0, -1.0, -1.0, -1.0, -1.0, -1.0, -1.0, -1.0, -1.0, -1.0, -1.0, -1.0, -1.0, -1.0, -1.0, -1.0, -1.0, -1.0, -1.0], [-1.0, -1.0, -1.0, -1.0, -1.0, -1.0, -1.0, -1.0, -1.0, -1.0, -1.0, -1.0, -1.0, -1.0, -1.0, -1.0, -1.0, -1.0, -1.0, -1.0, -1.0, -1.0, -1.0, -1.0, -1.0, -1.0, -1.0], [-1.0, -1.0, -1.0, -1.0, -1.0, -1.0, -1.0, -1.0, -1.0, -1.0, -1.0, -1.0, -1.0, -1.0, -1.0, -1.0, -1.0, -1.0, -1.0, -1.0, -1.0, -1.0, -1.0, -1.0, -1.0, -1.0, -1.0]], "Divider (kernel sum)"=sgl 10.0 ("Divider"), "error in (no error)"=w129, "Image Src"=w126) -> ("error out"=w139:errorcluster, "Image Dst Out"=w138:T9)  [unwired: 3 in, 3 out]
            n23 = case shown="\"Range 3\"" w110 {
              tunnel: ["Range 1 Templates - LEFT" "Range 0 Templates" "Range 2 Templates" "Range 3 Templates"] -> w171
              tunnel: [w537 w543 w554 w560] -> w169
              tunnel: [sgl 2.0 sgl 0.0 sgl 5.0 sgl 5.0] -> w168
              tunnel: [1 1 3 3] -> w167
              tunnel: [w534 w547 w550 w558] -> w112
              tunnel: "Correlation Score Threhsold" -> [w534 _ w550 w558]
              tunnel: "Correlation Score Threhsold (Range 0)" -> [_ w547 _ _]
              tunnel: [w531 w540 w549 w557] -> w107
              frame "Range 1", Default {
                w538 = TRUE
                w533 = FALSE
                n24 = Unbundle By Name("Range 1 Default\nSetting Values") -> ("Max Scale Diff\nfrom Main"=w531:dbl)
                n25 = Build Array(w533, w533, w533, w538, w538) -> (w537:bool[])
              }
              frame "Range 0" {
                (unwired) TRUE
                w544 = FALSE
                n26 = Unbundle By Name("Range 0 Default\nSetting Values") -> ("Max Scale Diff\nfrom Main"=w540:dbl)
                n27 = Build Array(w544, w544, w544, w544, w544) -> (w543:bool[])
              }
              frame "Range 2" {
                (unwired) FALSE
                w555 = TRUE
                n28 = Unbundle By Name("Range 2 Default\nSetting Values") -> ("Max Scale Diff\nfrom Main"=w549:dbl)
                n29 = Build Array(w555, w555, w555, w555, w555) -> (w554:bool[])
              }
              frame "Range 3" {
                (unwired) FALSE
                w561 = TRUE
                n30 = Unbundle By Name("Range 3 Default\nSetting Values") -> ("Max Scale Diff\nfrom Main"=w557:dbl)
                n31 = Build Array(w561, w561, w561, w561, w561) -> (w560:bool[])
              }
            }
            n32 = Unbundle(w171) -> ("Sub - 2 File Path"=w123:path, "Sub Beacon Template File Path - ARRAY"=w170:path[])
            n33 = call "pattern_match_subvi.vi"("Match Image In"=w138, "Settings"=w122, "Template Image In"=w121, "select (false=mod))"="select (true= use advanced features\nfase= dont use)", "ROI Descriptor"=w124, "error in (no error)"=w139, "Path In"=w123) -> ("Refnum out"=w118:T9, "Number of Matches"=w119:i32, "Matches"=w120:T13[], "error out"=w117:errorcluster)  [unwired: 5 in]
            n34 = Equal?(x=w119, y=1) -> (x = y?=w176:bool)
            n35 = Array To Cluster(array=w120) -> (cluster=w175:T14)
            n36 = Unbundle By Name(w175) -> ("Matches[0].Correlation Score"=w174:sgl)
            "Current Correlation Score" <- w174
            n37 = Greater?(x=w174, y=w112) -> (0:w173:bool)
            n38 = And(x=w176, y=w173) -> (x .and. y?=w172:bool)
            n39 = case shown="True" w172 {
              tunnel: w118 -> [w640 w668]
              tunnel: w168 -> [_ w670]
              tunnel: w169 -> [_ w669]
              tunnel: w117 -> [_ w667]
              tunnel: w122 -> [_ w666]
              tunnel: [w645 w653] -> w183
              tunnel: [w644 w665] -> w182
              tunnel: [w644 w664] -> w181
              tunnel: [w644 w655] -> w180
              tunnel: [w644 w663] -> w225
              tunnel: [w643 w651] -> w220
              tunnel: [w643 w652] -> w219
              tunnel: [w640 w662] -> w189
              tunnel: [w641 w658] -> w109
              tunnel: w175 -> [_ w661]
              tunnel: w170 -> [_ w660]
              tunnel: w110 -> [_ w659]
              tunnel: [w637 w657] -> w108
              tunnel: w107 -> [_ w650]
              frame False {
                w642 = 0.0
                w643 = sgl 0.0 ("Scale")
                # "Don't Move servo"
                n40 = Bundle(w642, w642) -> (w641:cluster{dbl, dbl})  [unwired: 1 in]
                n41 = Bundle(159.0, 119.0) -> (w637:cluster{dbl, dbl})  [unwired: 1 in]
                n42 = Initialize Array(FALSE, 5 ("dimension size")) -> (w645:bool[])
                n43 = Initialize Array(0.0, 5 ("dimension size")) -> (w644:dbl[])
              }
              frame True {
                n44 = Unbundle By Name(w661) -> ("Matches[0].Position"=w658:cluster{"x":sgl, "y":sgl}, "Matches[0].Bounding Box"=w671:cluster{"x":sgl, "y":sgl}[], "Matches[0].Scale"=w651:sgl, "Matches[0].Score"=w652:sgl)
                n45 = case shown="\"Range 1\", Default" w659 {
                  tunnel: w671 -> [w715 _]
                  tunnel: w670 -> [w711 _]
                  tunnel: w669 -> [w698 _]
                  tunnel: w668 -> [w696 w770]
                  tunnel: w667 -> [w695 _]
                  tunnel: w666 -> [w694 _]
                  tunnel: [w692 w779] -> w654
                  tunnel: [w691 w773] -> w665
                  tunnel: [w690 w774] -> w664
                  tunnel: [w689 w775] -> w655
                  tunnel: [w688 w776] -> w663
                  tunnel: w651 -> [w687 _]
                  tunnel: [w686 w770] -> w662
                  tunnel: w660 -> [w685 _]
                  tunnel: w651 -> [_ w771]
                  tunnel: [w684 w767] -> w657
                  tunnel: w658 -> [w684 _]
                  frame "Range 1", Default {
                    # "Build ROI for Individual Beacons Based on Main Bounding Box"
                    # "Starting X Lower Bound"
                    # "Beacons to Search For"
                    # "Length of\nIndividual Beacon ROI"
                    # "Length of Bounding Box"
                    # "Draw Bounding Box on Display Image"
                    n46 = Array To Cluster(array=w715) -> (cluster=w716:T15)
                    n47 = Unbundle By Name(w716) -> ("Bounding Box[0].x"=w709:sgl, "Bounding Box[0].y"=w705:sgl, "Bounding Box[2].x"=w712:sgl, "Bounding Box[2].y"=w704:sgl)
                    n48 = Bundle("x"=w709, "y"=w705, "x"=w712, "y"=w704) -> (w714:cluster{"x":sgl, "y":sgl, "x":sgl, "y":sgl})  [unwired: 1 in]
                    n49 = call "IMAQ Overlay Rectangle"("Rectangle"=w714, "Image"=w696) -> ("Image Out"=w693:T9)  [unwired: 8 in, 1 out]
                    n50 = Subtract(x=w712, y=w709) -> (x-y=w713:sgl)
                    n51 = Divide(x=w713, y=w711) -> (x/y=w710:sgl)
                    n52 = Multiply(x="Horiztonall Beacon \nCushion (pixels)", y=w687) -> (x*y=w706:sgl)
                    n53 = Divide(x=w706, y=sgl 100.0) -> (x/y=w701:sgl)
                    n54 = Subtract(x=w705, y=w701) -> (x-y=w703:sgl)
                    n55 = Add(x=w704, y=w701) -> (x+y=w702:sgl)
                    n56 = for {
                      N: 5 -> [_]
                      tunnel: w698 -> [w762] mode=indexing
                      shift-right: [w756] -> _
                      shift-left: w709 -> [w761]
                      tunnel: w710 -> [w760]
                      tunnel: w703 -> [w753]
                      tunnel: w702 -> [w752]
                      tunnel: [w759] -> w697 mode=indexing
                      tunnel: w701 -> [w754]
                      # "Divide Bounding Box"
                      # "Upper Bound of Current is\nLower Bound for Next"
                      n57 = case shown="True" w762 {
                        tunnel: w761 -> [w763 w764]
                        tunnel: w760 -> [_ w766]
                        tunnel: [w763 w765] -> w756
                        tunnel: [w763 w764] -> w758
                        frame False {
                          # "Don't Care"
                        }
                        frame True {
                          # "X Lower Bound"
                          n58 = Add(x=w764, y=w766) -> (x+y=w765:sgl)
                        }
                      }
                      n59 = Subtract(x=w758, y=w754) -> (x-y=w757:sgl)
                      n60 = Add(x=w756, y=w754) -> (x+y=w755:sgl)
                      n61 = call "Bound_RO_R_R0I.vi"("Bottom Right - Y"=w752, "Right - X"=w755, "Top Left - Y"=w753, "Top  Left - x"=w757) -> ("ROI Descriptor"=w759:T12)  [unwired: 7 in]
                    }
                    n62 = for {
                      N: 5 -> [_]
                      tunnel: w696 -> [w729]
                      tunnel: w695 -> [w728]
                      tunnel: w697 -> [w721] mode=indexing
                      tunnel: w685 -> [w727] mode=indexing
                      tunnel: [w726] -> w691 mode=indexing
                      tunnel: [w725] -> w690 mode=indexing
                      tunnel: [w724] -> w692 mode=indexing
                      tunnel: w698 -> [w723] mode=indexing
                      tunnel: w694 -> [w722]
                      shift-right: [w719] -> w686
                      shift-left: w693 -> [w720]
                      tunnel: [w718] -> w689 mode=indexing
                      tunnel: [w717] -> w688 mode=indexing
                      n63 = case shown="True" w723 {
                        tunnel: w729 -> [_ w744]
                        tunnel: w728 -> [_ w743]
                        tunnel: w721 -> [_ w742]
                        tunnel: w727 -> [_ w741]
                        tunnel: [w730 w737] -> w726
                        tunnel: [w730 w736] -> w725
                        tunnel: [FALSE w735] -> w724
                        tunnel: w722 -> [_ w734]
                        tunnel: [w730 w733] -> w718
                        tunnel: [w730 w732] -> w717
                        frame False {
                          w730 = sgl 0.0 ("x")
                        }
                        frame True {
                          n64 = call "Sub Beacon Pattern Match"("Image In"=w744, "ROI Descriptor (Geometric Matching 1)"=w742, "Settings (Geometric Matching 1)"=w734, "Template File Path (Geometric Matching 1)"=w741, "error in"=w743) -> ("Matches (Geometric Matching 1)"=w738:T13[], "Number of Matches (Geometric Matching 1)"=w739:i32)  [unwired: 19 in, 2 out]
                          n65 = Equal?(x=w739, y=1) -> (x = y?=w735:bool)
                          n66 = case shown="True" w735 {
                            tunnel: w738 -> [_ w750]
                            tunnel: [w745 w749] -> w737
                            tunnel: [w745 w748] -> w736
                            tunnel: [w745 w747] -> w733
                            tunnel: [w745 w746] -> w732
                            frame False {
                              w745 = sgl 0.0 ("x")
                            }
                            frame True {
                              n67 = Array To Cluster(array=w750) -> (cluster=w751:T16)
                              n68 = Unbundle By Name(w751) -> ("Matches (Geometric Matching 1)[0].Position.x"=w749:sgl, "Matches (Geometric Matching 1)[0].Position.y"=w748:sgl, "Matches (Geometric Matching 1)[0].Scale"=w747:sgl, "Matches (Geometric Matching 1)[0].Score"=w746:sgl)
                            }
                          }
                        }
                      }
                      n69 = call "IMAQ Overlay ROI"("ROI Descriptor"=w721, "Image"=w720) -> ("Image Out"=w719:T9)  [unwired: 8 in, 1 out]
                    }
                  }
                  frame "Range 0" {
                    w772 = sgl 0.0
                    w778 = FALSE
                    # "Don't Move servo"
                    # "Insert Current Scale into index 0"
                    n70 = Bundle(159.0, 119.0) -> (w767:cluster{dbl, dbl})  [unwired: 1 in]
                    n71 = Build Array(TRUE, w778, w778, w778, w778) -> (w779:bool[])
                    n72 = Build Array(w771, w772, w772, w772, w772) -> (w775:sgl[])
                    n73 = Build Array(w772, w772, w772, w772, w772) -> (w774:sgl[])
                    n74 = Build Array(w772, w772, w772, w772, w772) -> (w776:sgl[])
                    n75 = Build Array(w772, w772, w772, w772, w772) -> (w773:sgl[])
                  }
                }
                n76 = local read "History Size"() -> (w656:i32)
                n77 = for {
                  N: w656 -> [_]
                  tunnel: w651 -> [w675]
                  tunnel: w655 -> [w676] mode=indexing
                  tunnel: w654 -> [w674] mode=indexing
                  tunnel: [w673] -> w653 mode=indexing
                  tunnel: w650 -> [w672]
                  # "Check if Scale is within threshold of main,\ndsicard if not"
                  n78 = case shown="True" w674 {
                    selector: w674 -> [w677 _]
                    tunnel: w676 -> [_ w683]
                    tunnel: w675 -> [_ w682]
                    tunnel: [w677 w679] -> w673
                    tunnel: w672 -> [_ w678]
                    frame False {
                    }
                    frame True {
                      n79 = Subtract(x=w683, y=w682) -> (x-y=w681:sgl)
                      n80 = Absolute Value(x=w681) -> (abs(x)=w680:sgl)
                      n81 = Less?(x=w680, y=w678) -> (x < y?=w679:bool)
                    }
                  }
                }
              }
            }
            "Beacons Found" <- w183
            "X Coordinates" <- w182
            "Y Coordinates" <- w181
            "Beacon - Scales" <- w180
            "beacon - Scores" <- w225
            "Current  Scale" <- w220
            "Current  Score" <- w219
            n82 = shared-variable "RT myRIO Target - Overlord\\Localization_Variables_r0.lvlib\\RIGHT_BEACON_BOOL_array"(w183) -> ()  [unwired: 1 in, 1 out]
            n83 = shared-variable "RT myRIO Target - Overlord\\Localization_Variables_r0.lvlib\\RIGHT_BEACON_X_array"(w182) -> ()  [unwired: 1 in, 1 out]
            n84 = shared-variable "RT myRIO Target - Overlord\\Localization_Variables_r0.lvlib\\RIGHT_BEACON_Y_array"(w181) -> ()  [unwired: 1 in, 1 out]
            n85 = shared-variable "RT myRIO Target - Overlord\\Localization_Variables_r0.lvlib\\RIGHT_BEACON_Scales"(w180) -> ()  [unwired: 1 in, 1 out]
            n86 = Boolean To (0,1)(Boolean=w183) -> (0, 1=w227:i16[])
            n87 = Add Array Elements(numeric array=w227) -> (sum=w226:i16)
            n88 = Greater Or Equal?(x=w226, y=w167) -> (x >= y?=w158:bool)
            "Current Valid?" <- w158
            n89 = local read "History Size"() -> (w211:i32)
            n90 = Decrement(x=w211) -> (x-1=w224:i32)
            n91 = for {
              N: w211 -> [_]
              shift-right: [w615] -> w178
              shift-left: w223 -> [w603]
              tunnel: w224 -> [w611]
              shift-right: [w608] -> w146
              shift-left: w222 -> [w610]
              shift-right: [w607] -> w177
              shift-left: w221 -> [w609]
              tunnel: w220 -> [w606]
              tunnel: w219 -> [w605]
              tunnel: w158 -> [w604]
              i -> [w614]
              # "Reverse Index"
              n92 = Subtract(x=w611, y=w614) -> (x-y=w612:i32)
              n93 = Equal To 0?(x=w612) -> (x = 0?=w613:bool)
              n94 = case shown="True" w613 {
                tunnel: w612 -> [w616 w635]
                tunnel: w603 -> [w626 w628]
                tunnel: [w624 w627] -> w615
                tunnel: w604 -> [_ w636]
                tunnel: w610 -> [w621 w634]
                tunnel: w609 -> [w620 w633]
                tunnel: [w619 w631] -> w608
                tunnel: [w618 w632] -> w607
                tunnel: w606 -> [_ w630]
                tunnel: w605 -> [_ w629]
                frame False {
                  # "Shift Old"
                  n95 = Decrement(x=w616) -> (x-1=w617:i32)
                  n96 = Index Array(array=w626, index=w617) -> (element=w625:bool)
                  n97 = Index Array(array=w621, index=w617) -> (element=w623:dbl)
                  n98 = Index Array(array=w620, index=w617) -> (element=w622:dbl)
                  n99 = Replace Array Subset(array=w626, new element=w625, index=w616) -> (w624:bool[])
                  n100 = Replace Array Subset(array=w621, new element=w623, index=w616) -> (w619:dbl[])
                  n101 = Replace Array Subset(array=w620, new element=w622, index=w616) -> (w618:dbl[])
                }
                frame True {
                  # "Score"
                  # "Scale"
                  # "Valid"
                  # "insert New"
                  n102 = Replace Array Subset(array=w634, new element=w630, index=w635) -> (w631:dbl[])
                  n103 = Replace Array Subset(array=w633, new element=w629, index=w635) -> (w632:dbl[])
                  n104 = Replace Array Subset(array=w628, new element=w636, index=w635) -> (w627:bool[])
                }
              }
            }
            n105 = Boolean To (0,1)(Boolean=w178) -> (0, 1=w217:i16[])
            n106 = Add Array Elements(numeric array=w217) -> (sum=w216:i16)
            n107 = Greater Or Equal?(x=w216, y="Valid Treshold\nfor Lock") -> (x >= y?=w144:bool)
            "Lock Status" <- w144
            n108 = shared-variable "RT myRIO Target - Overlord\\Localization_Variables_r0.lvlib\\Image Lock - R"(w144) -> ()  [unwired: 1 in, 1 out]
            n109 = Initialize Array(u8 0, "Max Window\n for Avg") -> (w214:u8[])
            n110 = while {
              shift-right: [w586] -> w210
              shift-left: w214 -> [w588]
              tunnel: w178 -> [w594] mode=indexing
              shift-right: [w592] -> w207
              shift-left: u8 0 -> [w595]
              tunnel: w211 -> [w593]
              tunnel: "Max Window\n for Avg" -> [w585]
              i -> [w587]
              stop <- w589 stop-if-true
              # "Grab Last 'X' Valid Indexes"
              n111 = case shown="True" w594 {
                tunnel: w595 -> [w597 w599]
                tunnel: [w597 w602] -> w592
                tunnel: w588 -> [w596 w601]
                tunnel: w587 -> [_ w600]
                tunnel: [w596 w598] -> w586
                frame False {
                }
                frame True {
                  # "Update Index\nto use"
                  # "Increment\nValid Count"
                  n112 = Replace Array Subset(array=w601, new element=w600, index=w599) -> (w598:u8[])
                  n113 = Increment(x=w599) -> (x+1=w602:u8)
                }
              }
              n114 = Greater?(x=w587, y=w593) -> (0:w590:bool)
              n115 = Greater Or Equal?(x=w592, y=w585) -> (x >= y?=w591:bool)
              n116 = Or(x=w591, y=w590) -> (x .or. y?=w589:bool)
            }
            n117 = Greater Or Equal?(x=w207, y=u8 2) -> (x >= y?=w208:bool)
            n118 = case shown="True" w208 {
              tunnel: w207 -> [_ w569]
              tunnel: w210 -> [_ w575]
              tunnel: w146 -> [_ w574]
              tunnel: w177 -> [_ w573]
              tunnel: ["Avg Scale - Last" w567] -> w166
              tunnel: ["Avg Score - Last" w566] -> w165
              frame False {
              }
              frame True {
                w572 = 0.0
                n119 = for {
                  N: w569 -> [_]
                  tunnel: w575 -> [w582] mode=indexing
                  tunnel: w574 -> [w584]
                  tunnel: w573 -> [w583]
                  shift-right: [w580] -> w571
                  shift-left: w572 -> [w578]
                  shift-right: [w581] -> w570
                  shift-left: w572 -> [w577]
                  # "Fetch Last Valid Values"
                  n120 = Index Array(array=w584, index=w582) -> (element=w579:dbl)
                  n121 = Index Array(array=w583, index=w582) -> (element=w576:dbl)
                  n122 = Add(x=w579, y=w578) -> (x+y=w580:dbl)
                  n123 = Add(x=w576, y=w577) -> (x+y=w581:dbl)
                }
                n124 = To Double Precision Float(number=w569) -> (double precision float=w568:dbl)
                n125 = Divide(x=w571, y=w568) -> (x/y=w567:dbl)
                n126 = Divide(x=w570, y=w568) -> (x/y=w566:dbl)
                n127 = local write "Avg Scale - Last"(w567) -> ()
                n128 = local write "Avg Score - Last"(w566) -> ()
              }
            }
            "Avg Score" <- w165
            "Avg Scale" <- w166
            n129 = And(x=w144, y=w143) -> (x .and. y?=w145:bool)
            n130 = case shown="False" w145 {
              selector: w145 -> [_ w231]
              tunnel: [w229 w230] -> w142
              tunnel: w143 -> [w229 _]
              frame False {
              }
              frame True {
                # "Pull Down Start Up \nFlag"
                n131 = Not(x=w231) -> (.not. x?=w230:bool)
              }
            }
            n132 = Unbundle By Name(w122) -> ("Minimum Match Score"=w163:sgl, "Range Settings"=w194:T7[], "Curve Parameters"=w160:T6)
            n133 = Index Array(array=w194, index=u32 1) -> (element=w195:T7)
            n134 = Unbundle(w195) -> ("Min"=w162:dbl, "Max"=w161:dbl)  [unwired: 1 out]
            n135 = case shown="False" w142 {
              tunnel: w144 -> [w254 _]
              tunnel: w110 -> [w253 w530]
              tunnel: w166 -> [w252 _]
              tunnel: [w236 w530] -> w148
              tunnel: w166 -> [w251 _]
              tunnel: w165 -> [w250 _]
              tunnel: "Score\nCushion" -> [w249 _]
              tunnel: w163 -> [w248 w527]
              tunnel: w162 -> [w247 w526]
              tunnel: w161 -> [w246 w525]
              tunnel: w109 -> [w245 _]
              tunnel: w124 -> [w244 w529]
              tunnel: w160 -> [w243 _]
              tunnel: w160 -> [w242 w528]
              tunnel: [w241 w527] -> w152
              tunnel: [w240 w526] -> w150
              tunnel: [w239 w525] -> w151
              tunnel: [w238 w529] -> w149
              tunnel: [w237 w528] -> w157
              tunnel: [w235 FALSE] -> w159
              tunnel: w158 -> [w234 _]
              tunnel: w146 -> [w233 w523]
              tunnel: [w232 w523] -> w147
              frame False {
                # "Current Template"
                # "Image Lock?"
                n136 = case shown="True" w254 {
                  tunnel: w253 -> [w280 w322]
                  tunnel: [w280 w285] -> w236
                  tunnel: w252 -> [_ w323]
                  tunnel: w251 -> [_ w321]
                  tunnel: w250 -> [_ w319]
                  tunnel: w249 -> [_ w318]
                  tunnel: w248 -> [_ w317]
                  tunnel: w247 -> [_ w316]
                  tunnel: w246 -> [_ w315]
                  tunnel: w245 -> [_ w314]
                  tunnel: w244 -> [_ w313]
                  tunnel: w243 -> [_ w310]
                  tunnel: w242 -> [w258 w295]
                  tunnel: [w257 w290] -> w237
                  tunnel: [w269 w289] -> w238
                  tunnel: [w278 w288] -> w241
                  tunnel: [w277 w287] -> w240
                  tunnel: [w276 w286] -> w239
                  tunnel: [FALSE w284] -> w235
                  tunnel: w234 -> [_ w283]
                  tunnel: w233 -> [w255 w282]
                  tunnel: [w255 w281] -> w232
                  frame False {
                    # "Initial ROI Descriptor"
                    # "Check Other Camera?"
                    n137 = Unbundle By Name("No Lock Default\nSetting Values") -> ("Min Score"=w278:dbl, "Min Scale"=w277:dbl, "Max Scale"=w276:dbl, "Curve Parameters"=w259:T17)
                    n138 = Bundle(0, 0, 640, 480, 0) -> (w275:cluster{i32, i32, i32, i32, i32})  [unwired: 1 in]
                    n139 = call "IMAQ Convert Rectangle to ROI"("Rectangle"=w275) -> ("ROI Descriptor"=w269:T12)  [unwired: 8 in, 1 out]
                    n140 = Unbundle By Name(w259) -> ("Min Length"=w263:i32, "Row Search Step"=w264:i32, "Col Search Step"=w265:i32)
                    n141 = Unbundle(w258) -> ("Extraction Mode"=w260:u32, "Edge Threshold"=w261:i32, "Edge Filter Size"=w262:u32, "Max Endpoint Gap"=w266:i32, "Closed"=w267:bool, "Subpixel"=w268:bool)  [unwired: 3 out]
                    n142 = Bundle("Extraction Mode"=w260, "Edge Threshold"=w261, "Edge Filter Size"=w262, "Min Length"=w263, "Row Search Step"=w264, "Col Search Step"=w265, "Max Endpoint Gap"=w266, "Closed"=w267, "Subpixel"=w268) -> (w257:T18)  [unwired: 1 in]
                  }
                  frame True {
                    # "Update Search Settings"
                    # "Next State"
                    # "Changing Templates?"
                    # "Update Template"
                    n143 = case shown="\"Range 0\"" w322 {
                      selector: w322 -> [w455 w486 w504 w519]
                      tunnel: w323 -> [w456 w488 w505 w520]
                      tunnel: [w457 w487 w503 w518] -> w285
                      tunnel: [w471 w477 w497 w512] -> w320
                      tunnel: [w470 w476 w496 w511] -> w312
                      tunnel: [w469 w475 w495 w510] -> w311
                      tunnel: [w468 w478 w501 w516] -> w306
                      tunnel: [w467 w480 w498 w513] -> w298
                      tunnel: [w466 w481 w499 w514] -> w297
                      tunnel: [w465 w484 w500 w515] -> w296
                      frame "Range 1", Default {
                        # "Next Template"
                        # "Next Template"
                        n144 = local read "Range 1 Default\nSetting Values"() -> (w472:T1)
                        n145 = Unbundle By Name(w472) -> ("Lower Transition Scale"=w453:sgl, "Upper Transition Scale"=w454:sgl, "ROI Vertical"=w469:dbl, "ROI Horizontal"=w470:dbl, "Scale Cushion"=w471:dbl, "Curve Parameters"=w468:T17, "Min Score"=w467:dbl, "Min Scale"=w466:dbl, "Max Scale"=w465:dbl)
                        n146 = Less?(x=w456, y=w453) -> (x < y?=w464:bool)
                        n147 = Not(x=w464) -> (.not. x?=w463:bool)
                        n148 = Select(t=w455, s=w463, f=T4."Range 2" ("Initial Template 2")) -> (s? t:f=w460:T4)
                        n149 = Greater?(x=w456, y=w454) -> (0:w462:bool)
                        n150 = Not(x=w462) -> (.not. x?=w461:bool)
                        n151 = Select(t=w460, s=w461, f=T4."Range 0" ("Initial Template 2")) -> (s? t:f=w457:T4)
                      }
                      frame "Range 2" {
                        # "Next Template"
                        # "Next Template"
                        n152 = local read "Range 2 Default\nSetting Values"() -> (w485:T1)
                        n153 = Unbundle By Name(w485) -> ("Lower Transition Scale"=w483:sgl, "Upper Transition Scale"=w482:sgl, "ROI Vertical"=w475:dbl, "ROI Horizontal"=w476:dbl, "Scale Cushion"=w477:dbl, "Curve Parameters"=w478:T17, "Min Score"=w480:dbl, "Min Scale"=w481:dbl, "Max Scale"=w484:dbl)
                        n154 = Less?(x=w488, y=w483) -> (x < y?=w492:bool)
                        n155 = Not(x=w492) -> (.not. x?=w491:bool)
                        n156 = Select(t=w486, s=w491, f=T4."Range 3" ("Initial Template 2")) -> (s? t:f=w479:T4)
                        n157 = Greater?(x=w488, y=w482) -> (0:w490:bool)
                        n158 = Not(x=w490) -> (.not. x?=w489:bool)
                        n159 = Select(t=w479, s=w489, f=T4."Range 1" ("Initial Template 2")) -> (s? t:f=w487:T4)
                      }
                      frame "Range 3" {
                        # "Next Template"
                        n160 = local read "Range 3 Default\nSetting Values"() -> (w502:T1)
                        n161 = Unbundle By Name(w502) -> ("Upper Transition Scale"=w494:sgl, "ROI Vertical"=w495:dbl, "ROI Horizontal"=w496:dbl, "Scale Cushion"=w497:dbl, "Curve Parameters"=w501:T17, "Min Score"=w498:dbl, "Min Scale"=w499:dbl, "Max Scale"=w500:dbl)  [unwired: 1 out]
                        n162 = Greater?(x=w505, y=w494) -> (0:w507:bool)
                        n163 = Not(x=w507) -> (.not. x?=w506:bool)
                        n164 = Select(t=w504, s=w506, f=T4."Range 2" ("Initial Template 2")) -> (s? t:f=w503:T4)
                      }
                      frame "Range 0" {
                        # "Next Template"
                        n165 = local read "Range 0 Default\nSetting Values"() -> (w517:T1)
                        n166 = Unbundle By Name(w517) -> ("Lower Transition Scale"=w508:sgl, "ROI Vertical"=w510:dbl, "ROI Horizontal"=w511:dbl, "Scale Cushion"=w512:dbl, "Curve Parameters"=w516:T17, "Min Score"=w513:dbl, "Min Scale"=w514:dbl, "Max Scale"=w515:dbl)  [unwired: 1 out]
                        n167 = Less?(x=w520, y=w508) -> (x < y?=w522:bool)
                        n168 = Not(x=w522) -> (.not. x?=w521:bool)
                        n169 = Select(t=w519, s=w521, f=T4."Range 1" ("Initial Template 2")) -> (s? t:f=w518:T4)
                      }
                    }
                    n170 = Unbundle By Name(w306) -> ("Min Length"=w305:i32, "Row Search Step"=w304:i32, "Col Search Step"=w303:i32)
                    n171 = Unbundle(w310) -> ("Extraction Mode"=w309:u32, "Edge Threshold"=w308:i32, "Edge Filter Size"=w307:u32, "Max Endpoint Gap"=w302:i32, "Closed"=w301:bool, "Subpixel"=w300:bool)  [unwired: 3 out]
                    n172 = Bundle("Extraction Mode"=w309, "Edge Threshold"=w308, "Edge Filter Size"=w307, "Min Length"=w305, "Row Search Step"=w304, "Col Search Step"=w303, "Max Endpoint Gap"=w302, "Closed"=w301, "Subpixel"=w300) -> (w299:T18)  [unwired: 1 in]
                    n173 = Not Equal?(x=w285, y=w322) -> (x != y?=w284:bool)
                    n174 = case shown="True" w284 {
                      tunnel: w283 -> [w346 _]
                      tunnel: w321 -> [w345 _]
                      tunnel: w320 -> [w344 _]
                      tunnel: w319 -> [w343 _]
                      tunnel: w318 -> [w342 _]
                      tunnel: w317 -> [w341 _]
                      tunnel: w316 -> [w340 _]
                      tunnel: w315 -> [w339 _]
                      tunnel: w314 -> [w338 _]
                      tunnel: w313 -> [w337 _]
                      tunnel: w312 -> [w336 _]
                      tunnel: w311 -> [w335 _]
                      tunnel: [w333 w420] -> w288
                      tunnel: w299 -> [w324 _]
                      tunnel: [w332 w419] -> w287
                      tunnel: [w331 w418] -> w286
                      tunnel: w298 -> [_ _]
                      tunnel: w297 -> [_ _]
                      tunnel: w296 -> [_ _]
                      tunnel: w285 -> [_ w422]
                      tunnel: w295 -> [_ w435]
                      tunnel: [w325 w434] -> w290
                      tunnel: [w330 w429] -> w294
                      tunnel: [w329 w428] -> w293
                      tunnel: [w328 w411] -> w292
                      tunnel: [w327 w412] -> w291
                      tunnel: w282 -> [w326 w414]
                      tunnel: [w326 w413] -> w281
                      frame False {
                        w334 = 500.0 ("y")
                        # "Current Valid?"
                        # "********"
                        # "Apply Limit to Score"
                        # "Score out"
                        # "Apply Limits to ROI"
                        n175 = case shown="False" w346 {
                          tunnel: w343 -> [_ w395]
                          tunnel: w342 -> [_ w394]
                          tunnel: w345 -> [_ w385]
                          tunnel: w344 -> [w374 w393]
                          tunnel: [w357 w388] -> w330
                          tunnel: [w356 w384] -> w329
                          tunnel: [w355 w387] -> w328
                          tunnel: [w354 w386] -> w327
                          tunnel: [w370 w383] -> w347
                          tunnel: [w369 w382] -> w332
                          tunnel: [w368 w381] -> w331
                          tunnel: w337 -> [w366 _]
                          tunnel: w341 -> [w353 _]
                          tunnel: w340 -> [w352 _]
                          tunnel: w339 -> [w351 _]
                          tunnel: w338 -> [_ w380]
                          tunnel: w336 -> [_ w376]
                          tunnel: w335 -> [_ w377]
                          tunnel: [w349 w375] -> w325
                          tunnel: w324 -> [w349 w375]
                          frame False {
                            # "Current Match was Invalid"
                            n176 = Divide(x=w374, y=sgl 3.0) -> (x/y=w372:dbl)
                            n177 = Subtract(x=w352, y=w372) -> (x-y=w369:dbl)
                            n178 = Add(x=w351, y=w372) -> (x+y=w368:dbl)
                            n179 = Subtract(x=w353, y="Score Decay \nFactor 2") -> (x-y=w370:dbl)
                            n180 = call "IMAQ Convert ROI to Rectangle"("ROI Descriptor"=w366) -> ("Rectangle"=w367:T19)  [unwired: 8 in, 1 out]
                            n181 = Unbundle By Name(w367) -> ("Left"=w361:i32, "Top"=w360:i32, "Right"=w359:i32, "Bottom"=w358:i32)
                            n182 = To Long Integer(number="ROI Decay Factor (px)") -> (32bit integer=w363:i32)
                            n183 = Divide(x="ROI Decay Factor (px)", y=sgl 10.0) -> (x/y=w365:dbl)
                            n184 = Subtract(x=w361, y=w363) -> (x-y=w357:i32)
                            n185 = Add(x=w359, y=w363) -> (x+y=w355:i32)
                            n186 = To Long Integer(number=w365) -> (32bit integer=w362:i32)
                            n187 = Subtract(x=w360, y=w362) -> (x-y=w356:i32)
                            n188 = Add(x=w358, y=w362) -> (x+y=w354:i32)
                          }
                          frame True {
                            (unwired) sgl 109.0 ("x")
                            (unwired) sgl 159.0 ("x")
                            # "Current Match was Valid"
                            # "Center of Image"
                            # "Main ROI"
                            # "Horizontal Scale \n(smaller number = smaller ROI)"
                            n189 = Subtract(x=w395, y=w394) -> (x-y=w383:dbl)
                            n190 = case shown="0, Default" "ROBOT STATE\n(fwd, bwd, neither) 2" {
                              tunnel: w385 -> [w400 w405 w410]
                              tunnel: [w399 w401 w406] -> w381
                              tunnel: w393 -> [w397 w404 w409]
                              tunnel: [w398 w402 w407] -> w382
                              frame 0, Default {
                                n191 = Subtract(x=w400, y=w397) -> (x-y=w398:dbl)
                                n192 = Add(x=w397, y=w400) -> (x+y=w399:dbl)
                              }
                              frame 1 {
                                n193 = Subtract(x=w405, y=5.0) -> (x-y=w402:dbl)
                                n194 = Add(x=w404, y=w405) -> (x+y=w401:dbl)
                              }
                              frame -1 {
                                n195 = Subtract(x=w410, y=w409) -> (x-y=w407:dbl)
                                n196 = Add(x=5.0 ("y"), y=w410) -> (x+y=w406:dbl)
                              }
                            }
                            n197 = Unbundle(w380) -> ("x"=w379:dbl, "y"=w378:dbl)
                            n198 = Divide(x=w385, y=w377) -> (x/y=w391:dbl)
                            n199 = Multiply(x=w385, y=w376) -> (x*y=w389:dbl)
                            n200 = Divide(x=w389, y=sgl 2.0) -> (x/y=w392:dbl)
                            n201 = Add(x=w378, y=w391) -> (x+y=w386:dbl)
                            n202 = Subtract(x=w378, y=w391) -> (x-y=w384:dbl)
                            n203 = Subtract(x=w379, y=w392) -> (x-y=w388:dbl)
                            n204 = Add(x=w392, y=w379) -> (x+y=w387:dbl)
                          }
                        }
                        n205 = Greater?(x=w347, y=w334) -> (0:w348:bool)
                        n206 = Select(t=w347, s=w348, f=w334) -> (s? t:f=w333:dbl)
                      }
                      frame True {
                        w415 = 80.0 ("Avg Scale - Last")
                        w425 = sgl 125.0 ("x")
                        w426 = sgl 109.0 ("x")
                        w427 = sgl 159.0 ("x")
                        # "Reset Scale to 100"
                        # "\"Start Scale\""
                        # "Center of Image"
                        # "Main ROI"
                        # "Horizontal Scale \n(smaller number = smaller ROI)"
                        # "Apply New Curve Parameters"
                        # "Next State"
                        # "Changing States - Apply Initial Settings for that State"
                        n207 = local read "History Size"() -> (w416:i32)
                        n208 = case shown="\"Range 1\", Default" w422 {
                          tunnel: [w449 w450 w451 w452] -> w421
                          frame "Range 1", Default {
                            n209 = local read "Range 1 Default\nSetting Values"() -> (w449:T1)
                          }
                          frame "Range 2" {
                            n210 = local read "Range 2 Default\nSetting Values"() -> (w450:T1)
                          }
                          frame "Range 3" {
                            n211 = local read "Range 3 Default\nSetting Values"() -> (w451:T1)
                          }
                          frame "Range 0" {
                            n212 = local read "Range 0 Default\nSetting Values"() -> (w452:T1)
                          }
                        }
                        n213 = for {
                          N: w416 -> [_]
                          tunnel: w415 -> [w446]
                          shift-right: [w445] -> w413
                          shift-left: w414 -> [w448]
                          i -> [w447]
                          n214 = Replace Array Subset(array=w448, new element=w446, index=w447) -> (w445:dbl[])
                        }
                        n215 = local write "Avg Scale - Last"(w415) -> ()
                        n216 = Unbundle By Name(w421) -> ("Min Score"=w420:dbl, "Min Scale"=w419:dbl, "Max Scale"=w418:dbl, "Curve Parameters"=w417:T17, "ROI Vertical"=w424:dbl, "ROI Horizontal"=w423:dbl)
                        n217 = Unbundle By Name(w417) -> ("Min Length"=w439:i32, "Row Search Step"=w440:i32, "Col Search Step"=w441:i32)
                        n218 = Unbundle(w435) -> ("Extraction Mode"=w436:u32, "Edge Threshold"=w437:i32, "Edge Filter Size"=w438:u32, "Max Endpoint Gap"=w442:i32, "Closed"=w443:bool, "Subpixel"=w444:bool)  [unwired: 3 out]
                        n219 = Bundle("Extraction Mode"=w436, "Edge Threshold"=w437, "Edge Filter Size"=w438, "Min Length"=w439, "Row Search Step"=w440, "Col Search Step"=w441, "Max Endpoint Gap"=w442, "Closed"=w443, "Subpixel"=w444) -> (w434:T18)  [unwired: 1 in]
                        n220 = Divide(x=w425, y=w424) -> (x/y=w432:dbl)
                        n221 = Multiply(x=w425, y=w423) -> (x*y=w430:dbl)
                        n222 = Divide(x=w430, y=sgl 2.0) -> (x/y=w433:dbl)
                        n223 = Add(x=w426, y=w432) -> (x+y=w412:dbl)
                        n224 = Subtract(x=w426, y=w432) -> (x-y=w428:dbl)
                        n225 = Subtract(x=w427, y=w433) -> (x-y=w429:dbl)
                        n226 = Add(x=w433, y=w427) -> (x+y=w411:dbl)
                      }
                    }
                    n227 = call "Bound_RO_R_R0I.vi"("Bottom Right - Y"=w291, "Right - X"=w292, "Top Left - Y"=w293, "Top  Left - x"=w294) -> ("ROI Descriptor"=w289:T12)  [unwired: 7 in]
                  }
                }
              }
              frame True {
              }
            }
            "Next Template" <- w148
            n228 = Less?(x=w152, y="Absolute\nMinimum Score") -> (x < y?=w200:bool)
            n229 = Less?(x=w150, y="Absolute\nMinimum Scale") -> (x < y?=w203:bool)
            n230 = Greater?(x=w151, y="Absolute\nMaximum Scale") -> (0:w206:bool)
            n231 = Greater?(x=w150, y=w151) -> (0:w202:bool)
            n232 = Less?(x=w151, y=w150) -> (x < y?=w205:bool)
            n233 = Select(t="Absolute\nMinimum Score", s=w200, f=w152) -> (s? t:f=w188:dbl)
            "New Min Score" <- w188
            n234 = Or(x=w203, y=w202) -> (x .or. y?=w201:bool)
            n235 = Or(x=w206, y=w205) -> (x .or. y?=w204:bool)
            n236 = Select(t="Absolute\nMinimum Scale", s=w201, f=w150) -> (s? t:f=w187:dbl)
            "New Low Scale" <- w187
            n237 = Select(t="Absolute\nMaximum Scale", s=w204, f=w151) -> (s? t:f=w186:dbl)
            "New high Scale" <- w186
            n238 = Bundle("index"=w193, "Min"=w187, "Max"=w186) -> (w192:cluster{"index":u32, "Min":dbl, "Max":dbl})  [unwired: 1 in]
            n239 = Replace Array Subset(array=w194, new element=w192, index=w193) -> (w191:T7[])
            n240 = Bundle By Name(cluster=w122, "Minimum Match Score"=w188, "Range Settings"=w191, "Curve Parameters"=w157) -> (w190:T8)
            n241 = call "IMAQ Overlay ROI"("ROI Descriptor"=w149, "Image"=w189) -> ("Image Out"=→"Right Image out":T9)  [unwired: 8 in, 1 out]
            n242 = Unbundle By Name(w157) -> ("Min Length"=w156:i32, "Row Search Step Size"=w155:i32, "Col Search Step Size"=w154:i32)
            n243 = Bundle("Min Length"=w156, "Row Search Step Size"=w155, "Col Search Step Size"=w154) -> (w153:T20)  [unwired: 1 in]
            n244 = Bundle("Min Score"=w188, "Min"=w187, "Max"=w186, w153) -> (w185:T21)  [unwired: 1 in]
            n245 = case shown="True" w159 {
              tunnel: w108 -> [w782 w788]
              tunnel: w158 -> [w783 w794]
              tunnel: w183 -> [_ _]
              tunnel: w185 -> [w785 w792]
              tunnel: w144 -> [w784 w795]
              tunnel: w148 -> [w781 w793]
              tunnel: [w780 w791] -> w141
              frame False {
                n246 = Bundle(w784, w783, "Initial Template"=w781, "Position"=w782, w785) -> (w780:T22)  [unwired: 1 in]
              }
              frame True {
                # "Check if Tracking is Available for the Next Template State"
                n247 = local read "Current Template"() -> (w786:T4)
                n248 = Unbundle(w788) -> ("x"=w790:dbl, "y"=w789:dbl)
                n249 = case shown="\"Range 1\"" w793 {
                  tunnel: w790 -> [w800 w809 _ _]
                  tunnel: w789 -> [w796 w808 _ _]
                  tunnel: w788 -> [_ w806 w817 _]
                  tunnel: [w799 w807 w817 w820] -> w787
                  tunnel: w786 -> [w797 w805 _ _]
                  frame "Range 1" {
                    n250 = case shown="\"Range 2\"" w797 {
                      tunnel: w800 -> [w801 w804]
                      tunnel: [w801 w802] -> w798
                      frame "Range 0", Default {
                      }
                      frame "Range 2" {
                        n251 = Add(x=w804, y=70.0) -> (x+y=w802:dbl)
                      }
                    }
                    n252 = Bundle("x"=w798, "y"=w796) -> (w799:cluster{"x":dbl, "y":dbl})  [unwired: 1 in]
                  }
                  frame "Range 2" {
                    # "Depends on Current State"
                    n253 = case shown="\"Range 1\"" w805 {
                      tunnel: w809 -> [w814 _ _]
                      tunnel: w808 -> [w811 _ _]
                      tunnel: [w810 w815 w816] -> w807
                      tunnel: w806 -> [_ w815 w816]
                      frame "Range 1" {
                        n254 = Add(x=w814, y=-70.0) -> (x+y=w812:dbl)
                        n255 = Bundle(w812, "y"=w811) -> (w810:cluster{dbl, "y":dbl})  [unwired: 1 in]
                      }
                      frame "Range 2", Default {
                      }
                      frame "Range 3" {
                      }
                    }
                  }
                  frame "Range 3", Default {
                  }
                  frame "Range 0" {
                    # "Don't Move servo"
                    n256 = Bundle(159.0, 119.0) -> (w820:cluster{dbl, dbl})  [unwired: 1 in]
                  }
                }
                n257 = Bundle(w795, w794, "Initial Template"=w793, "Position"=w787, w792) -> (w791:T22)  [unwired: 1 in]
              }
            }
            "Tracking Info" <- w141
            n258 = shared-variable "RT myRIO Target - Overlord\\Localization_Variables_r0.lvlib\\Info - Right"(w141) -> ()  [unwired: 1 in, 1 out]
          }
          frame #2 {
            n259 = shared-variable "RT myRIO Target - Overlord\\Localization_Variables_r0.lvlib\\Right Servo Angle_Image"(w823) -> ()  [unwired: 1 in, 1 out]
            n260 = shared-variable "RT myRIO Target - Overlord\\Localization_Variables_r0.lvlib\\RIGHT_FLAG"(TRUE ("RIGHT_FLAG")) -> ()  [unwired: 1 in, 1 out]
          }
        }
        "Startup Flag" <- w75
        "Valid Scale History" <- w82
        "Valid Beacon History - in" <- w84
        "Valid Score History" <- w81
        "Current Search Settings" <- w92
        "Current Template" <- w79
      }
    }
    frame #2 {
      n261 = call <vilib>:"IMAQdx Close Camera.vi"("Session In"=w825) -> ()  [unwired: 10 in, 1 out]
    }
  }
